vi "Main_v4_OJ.vi"() -> ()   [LabVIEW 2023]
uses:
  AD2_MSO_SDK_class/MSOConfig.ctl
  AD2_MSO_SDK_class/AD2TriggerSources.ctl
  AD2_MSO_SDK_class/MSORangeCh.ctl
  AD2_DO_SDK_class/DOConfigureCustomData.ctl
  AD2_DO_SDK_class/DOTrigger.ctl
  AD2_WFG_SDK_class/AD2TriggerSources.ctl
  AD2_DO_SDK_class/DOCustomData.ctl
  Application_class/Application.lvclass
  <vilib>/Utility/error.llb/Error Cluster From Error Code.vi
  <vilib>/ErrorRing/Error Ring.xnode
  AD2_SDK_class/AD2_SDK.lvclass
  AFG3022B_OJ_class/AFG3022B_OJ.lvclass
  Experiment_class/Experiment.lvclass
  TDMSLogger__class/TDMSLogger_class/TDMSLogger.lvclass
  CetoniPump_class/CetoniPump.lvclass
  TBS2000Series_class/TBS2000Series.lvclass
  TC0608_class/TC0608.lvclass
  AD2_DO_SDK_class/AD2_DO_SDK.lvclass
  AD2_MSO_SDK_class/AD2_MSO_SDK.lvclass
panel:
  out "Pump Status":T1(array[cluster])
  in  "Tab Control":T2(tab)=enum."InstrumentTests"
  in  "Cetoni Pump":bool
  in  "Initialize selected Instruments":bool
  in  "Peltier Controller":bool
  in  "Analog Discovery":bool
  in  "Function Generator":bool
  in  "Device Configuration Folder":string="C:\\Users\\Public\\Documents\\QmixElements\\Projects\\default_project\\Configurations\\sinle"
  in  "Peltier VISA resource name":refnum<visa-resource-name>
  in  "VISA resource name":refnum<visa-resource-name>
  in  "Change Freq Ch1 (Hz)":dbl
  in  "Enable Channels":cluster{"Ch1":bool, "Ch2":bool}
  in  "Oscilloscope Test":cluster{"Source Main":i32, "Source Probe":i32}={"Source Main"=2, "Source Probe"=1} {"Source Probe" items=["Math", "Channel 1", "Channel 2", "Channel 3", "Channel 4"]; "Source Main" items=["Math", "Channel 1", "Channel 2", "Channel 3", "Channel 4"]}
  in  "ReadOscilloscopeChannel":bool
  out "Temperature (C)":dbl
  in  "Read Peltier":bool
  in  "Image  Aquisition":T3={"Minimum Time between frames(s)"=10.0, "Number of Frames"=0} {"Minimum Time between frames(s)" min=0.005}
  in  "Take Images":bool
  in  "Pump: GoToLevel":bool
  in  "GoToLevelSettings":T4
  in  "refill below level":dbl=1000.0
  in  "Timeout Refill":dbl=20.0 caption="Time Target (s)"
  in  "Pump: CheckLevel&Refill":bool
  in  "Pump: Reference Move":bool
  in  "Pump: Refill":bool
  in  "Index":i32
  in  "Pump: Empty":bool
  in  "Pump: Read Status":bool
  in  "SyringeSettings":T5={"Maximum Piston Stroke (mm)"=100.0, "Inner Diameter (mm)"=12.0}
  in  "index configure syringe":i32
  in  "Pump: Configure":bool
  in  "Pump: STOP":bool
  in  "Source (1: Channel 1)":i32(ring)=1 items=["Math", "Channel 1", "Channel 2", "Channel 3", "Channel 4"]
  out "Peak-to-Peak":dbl format="%.2p"
  out "Frequency":dbl format="%.2p"
  in  "MeasurePowerOsc":bool
  out "Oscilloscope Results Test":T6 {"Probe Current" format="%.2p"; "Phase Angle" format="%.2p"; "Main Freq" format="%.2p"; "Main Volt" format="%.2p"}
  in  "milliseconds to wait 2":u32
  in  "Refill Rate(ul/min)":dbl=10000.0
  in  "Function Generator":T7
  in  "Change Amplitude Ch1(V)":dbl min=0.0 max=10.0
  in  "Wait After cond Refill":dbl
  in  "Start Experiment":bool
  in  "List of Frequencies":dbl[](array[numeric]) min=0.001
  in  "List of Amplitudes":dbl[](array[numeric]) min=0.001
  in  "List of Flow rates":dbl[](array[numeric])
  out "Total Number of Commands in Experiment":i32
  out "Commands Left in Experiment":i32
  out "Experiment Progress (%)":dbl
  in  "Number of Images at each frequency":i32
  in  "wait after frequency change (s)":dbl
  in  "wait between frames (s)":dbl
  in  "Freq Start":dbl
  in  "Freq Increment":dbl
  in  "Number of Frequencies":i32
  in  "FIll Frequency List":bool
  out "LOG":string
  in  "Time To wait":dbl
  in  "Wait":bool
  in  "Configure MSO":bool
  in  "MSO":T8={"Timing"={"Enable"=TRUE, "Samples In"=100000.0, "Sample Rate"=1250000.0, "Mode"=enum."Single Sample"}, "Trigger"={"Hysteresis"=0.0, "Trigger Level"=0.0, "Trigger Condition"=0, "Trigger Type"=0, "Trigger Channel"=0, "secTimeout"=1.0, "TrigrSrc"=enum."trigrsrcNone"}, "Range Ch1"={"idxChannel"=0, "voltOffset"=0.0, "VoltsRange"=50}, "Range Ch 2"={"idxChannel"=1, "voltOffset"=0.0, "VoltsRange"=50}} {"Range Ch 2"."VoltsRange" items=["High 50V"=50, "Low5V"=5]; "Range Ch1"."VoltsRange" items=["High 50V"=50, "Low5V"=5]; "Trigger"."Trigger Channel" items=["Channel 1"=0, "Channel 2"=1, "Both"=-1]; "Trigger"."Trigger Type" items=["Edge", "Pulse", "Transition"]; "Trigger"."Trigger Condition" items=["Rising", "Falling"]}
  in  "Read MSO":bool
  out "Waveform Graph":waveform(dbl)[](graph)
  out "Power (W)":dbl format="%0.2p"
  out "Impedance":dbl
  out "Phase (deg)":dbl
  in  "MeasurePower":bool
  in  "Trigg AD2":bool
  in  "Configure DO":bool
  in  "?":T11={"DO Trigger"={"secRun(0=Cont)"=0.0, "secWait"=0.0, "cRepeat(0=inf)"=0, "Repeat Trigger"=TRUE, "TrigrSrc"=enum."trigsrcPC"}, "CustomData"=[{"Data"=[FALSE, TRUE, FALSE, FALSE, FALSE, FALSE, FALSE, FALSE, FALSE, FALSE, FALSE, FALSE, FALSE, FALSE, FALSE, FALSE, FALSE, FALSE, FALSE, FALSE, FALSE, FALSE], "Freq"=1000.0, "#Bits"=100, "Enable"=TRUE, "IdleState"=0}, {"Data"=[], "Freq"=0.0, "#Bits"=0, "Enable"=FALSE, "IdleState"=0}, {"Data"=[], "Freq"=0.0, "#Bits"=0, "Enable"=FALSE, "IdleState"=0}, {"Data"=[], "Freq"=0.0, "#Bits"=0, "Enable"=FALSE, "IdleState"=0}, {"Data"=[], "Freq"=0.0, "#Bits"=0, "Enable"=FALSE, "IdleState"=0}, {"Data"=[], "Freq"=0.0, "#Bits"=0, "Enable"=FALSE, "IdleState"=0}, {"Data"=[], "Freq"=0.0, "#Bits"=0, "Enable"=FALSE, "IdleState"=0}, {"Data"=[], "Freq"=0.0, "#Bits"=0, "Enable"=FALSE, "IdleState"=0}, {"Data"=[], "Freq"=0.0, "#Bits"=0, "Enable"=FALSE, "IdleState"=0}, {"Data"=[], "Freq"=0.0, "#Bits"=0, "Enable"=FALSE, "IdleState"=0}, {"Data"=[], "Freq"=0.0, "#Bits"=0, "Enable"=FALSE, "IdleState"=0}, {"Data"=[], "Freq"=0.0, "#Bits"=0, "Enable"=FALSE, "IdleState"=0}, {"Data"=[], "Freq"=0.0, "#Bits"=0, "Enable"=FALSE, "IdleState"=0}, {"Data"=[FALSE, FALSE, FALSE, FALSE, FALSE, FALSE, FALSE, FALSE, FALSE, FALSE, FALSE, FALSE, FALSE, FALSE, FALSE, FALSE, FALSE, FALSE, FALSE, FALSE, FALSE, FALSE, FALSE], "Freq"=0.0, "#Bits"=0, "Enable"=FALSE, "IdleState"=0}, {"Data"=[FALSE, FALSE, FALSE, FALSE, FALSE, FALSE, FALSE, FALSE, FALSE, FALSE, FALSE, FALSE, FALSE, FALSE, FALSE, FALSE, FALSE, FALSE, FALSE, FALSE, FALSE, FALSE, FALSE], "Freq"=0.0, "#Bits"=0, "Enable"=FALSE, "IdleState"=0}]}
  in  "ABORT":bool
  out "Status":string="Program Started\nPlease connect to instruments"
  out "error out":errorcluster
  in  "Exit":bool
  # "Notes: \nChange frequency input to MHz\ninvestigate index in GoToLevelSettings, might be unneccesary"
  # "Peltier"
  # "Camera"
  # "Pump"
  # "Function Generator"
  # "Oscilloscope"
  # "Choose this carefully!\nYou can probably set this one low, since reading the peltier is slow. You might get problems when you start streaming images to HDD.\nThe program doesnt know when the camera is ready to aquire a new image. For large experiments you cannot store all images in RAM"
  # "The Pump will use index 0 for experiments\nPlease put your syringe here"
  # "Change Flow Rate\nChange Amplitude\nChange Frequency\nConditional Refill and wait\nEnable FG ch1\nWait\nRecord N times\nDisable Ch1\nWait\nRecord N times"
  # "Connect Ch1 to Piezo\nConnect Ch2 to voltage probe\nSet VoltsRange to LOW on ch2"
  # "Not sure if this is needed if we read the oscilloscope manually instead"
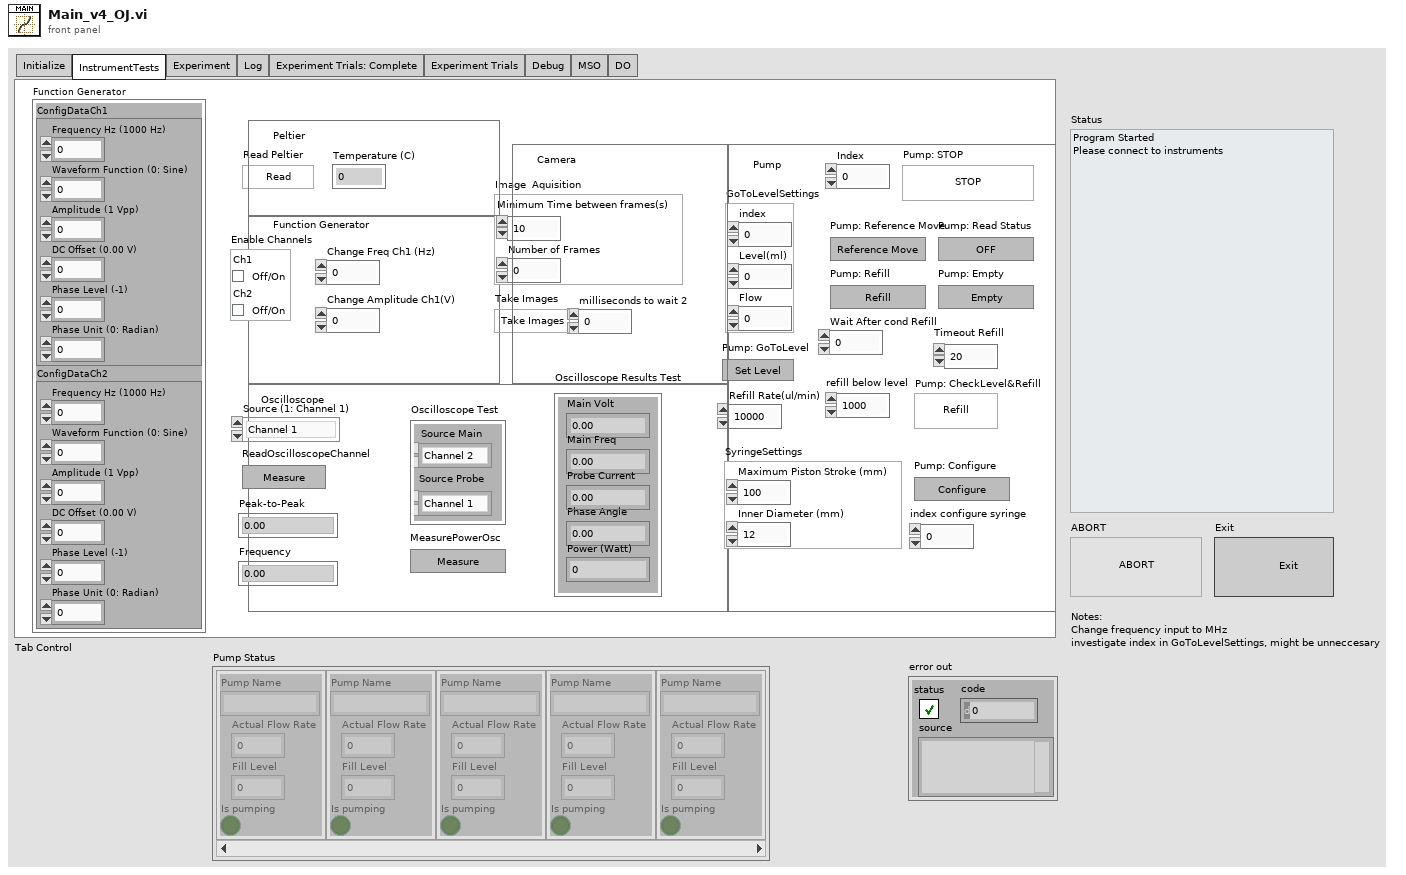
[diagram p1: front panel]
types:
  T1 = cluster{"Pump Name":string, "Actual Flow Rate":dbl, "Fill Level":dbl, "Is pumping":bool}[]
  T2 = enum32{"Initialize", "InstrumentTests", "Experiment", "Log", "Experiment Trials: Complete", "Experiment Trials", "Debug", "MSO", "DO"}
  T3 = cluster{"Minimum Time between frames(s)":dbl, "Number of Frames":i32}
  T4 = cluster{"index":i32, "Level(ml)":dbl, "Flow":dbl}
  T5 = cluster{"Maximum Piston Stroke (mm)":dbl, "Inner Diameter (mm)":dbl}
  T6 = cluster{"Main Volt":dbl, "Main Freq":dbl, "Phase Angle":dbl, "Probe Current":dbl, "Power (Watt)":dbl}
  T7 = cluster{"ConfigDataCh1":cluster{"Frequency Hz (1000 Hz)":dbl, "Waveform Function (0: Sine)":u16, "Amplitude (1 Vpp)":dbl, "DC Offset (0.00 V)":dbl, "Phase Level (-1)":dbl, "Phase Unit (0: Radian)":u16}, "ConfigDataCh2":cluster{"Frequency Hz (1000 Hz)":dbl, "Waveform Function (0: Sine)":u16, "Amplitude (1 Vpp)":dbl, "DC Offset (0.00 V)":dbl, "Phase Level (-1)":dbl, "Phase Unit (0: Radian)":u16}}
  T8 = typedef "AD2_MSO_SDK.lvclass/MSOConfig.ctl" = cluster{"Timing":cluster{"Enable":bool, "Samples In":dbl, "Sample Rate":dbl, "Mode":enum16{"Single Sample", "Scanshift", "Multiple Samples", "Scan Screen"}}, "Trigger":cluster{"Hysteresis":dbl, "Trigger Level":dbl, "Trigger Condition":i32, "Trigger Type":i32, "Trigger Channel":i32, "secTimeout":dbl, "TrigrSrc":T9}, "Range Ch1":T10, "Range Ch 2":T10}
  T9 = typedef "AD2_MSO_SDK.lvclass/AD2TriggerSources.ctl" = enum8{"trigrsrcNone", "trigsrcPC", "trigsrcDetectorAnalogIn", "trigsrcDetectorDigitalIn", "trigsrcAnalogIn", "trigsrcDigitalIn", "trigsrcDigitalOut", "trigsrcAnalogOut1", "trigsrcAnalogOut2", "trigsrcAnalogOut3", "trigsrcAnalogOut4", "trigsrcExternal1", "trigsrcExternal2", "trigsrcExternal3", "trigsrcExternal4", ""}
  T10 = typedef "AD2_MSO_SDK.lvclass/MSORangeCh.ctl" = cluster{"idxChannel":i32, "voltOffset":dbl, "VoltsRange":u16}
  T11 = typedef "DOConfigureCustomData.ctl" = cluster{"DO Trigger":T12, "CustomData":T14}
  T12 = typedef "AD2_DO_SDK.lvclass/DOTrigger.ctl" = cluster{"secRun(0=Cont)":dbl, "secWait":dbl, "cRepeat(0=inf)":i32, "Repeat Trigger":bool, "TrigrSrc":T13}
  T13 = typedef "AD2_SDK.lvclass/AD2TriggerSources.ctl" = enum8{"trigrsrcNone", "trigsrcPC", "trigsrcDetectorAnalogIn", "trigsrcDetectorDigitalIn", "trigsrcAnalogIn", "trigsrcDigitalIn", "trigsrcDigitalOut", "trigsrcAnalogOut1", "trigsrcAnalogOut2", "trigsrcAnalogOut3", "trigsrcAnalogOut4", "trigsrcExternal1", "trigsrcExternal2", "trigsrcExternal3", "trigsrcExternal4", ""}
  T14 = typedef "AD2_DO_SDK.lvclass/DOCustomData.ctl" = cluster{"Data":bool[], "Freq":dbl, "#Bits":u32, "Enable":bool, "IdleState":u16}[]
  T15 = cluster{"Minimum Time between frames":dbl, "Number of Frames":i32}
  T16 = cluster{"Pump Handle":i64, "Pump Name":string, "Maximum Volume":dbl, "Maximum Flow Rate":dbl, "Flow Rate":dbl, "Target Level":dbl, "Valve Handle":i64, "Has Valve?":bool, "Actual valve position":i32}[]
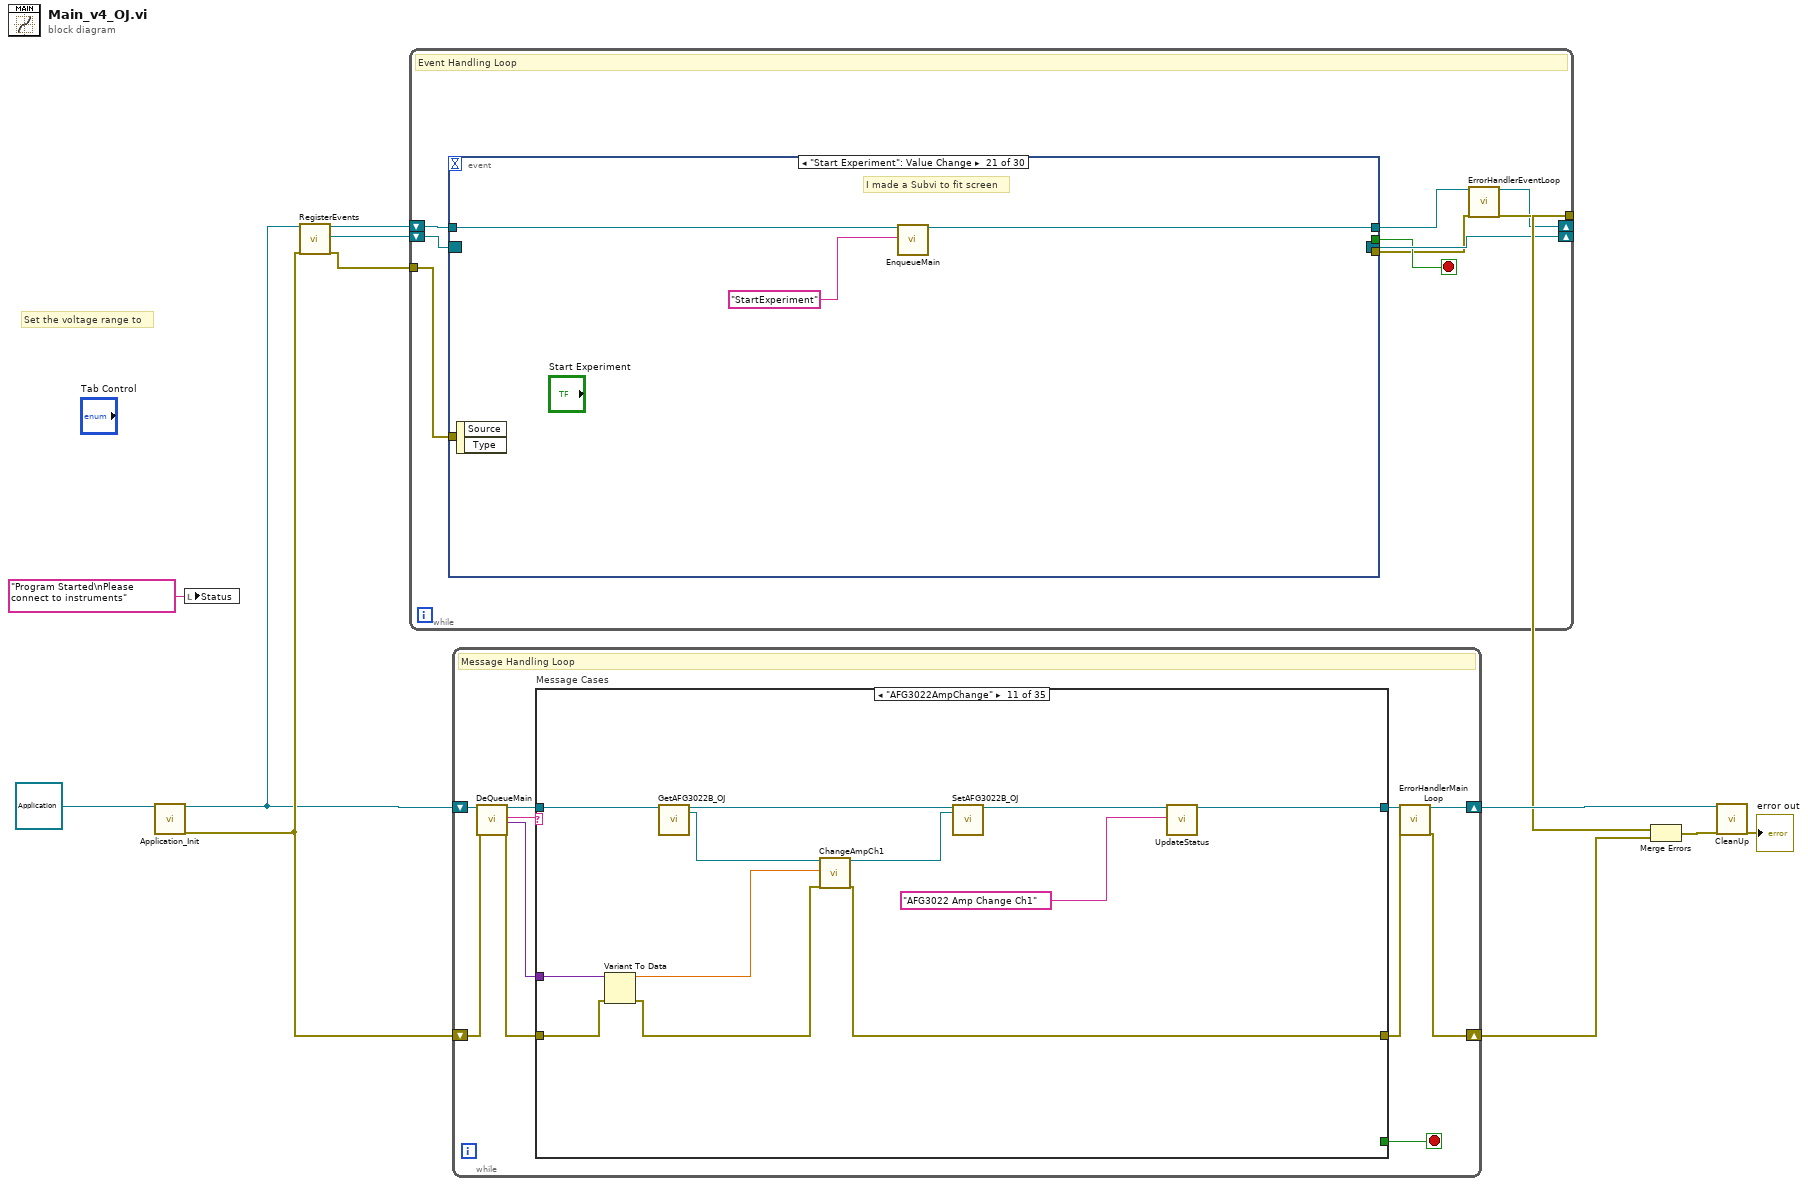
[diagram p0: block diagram]
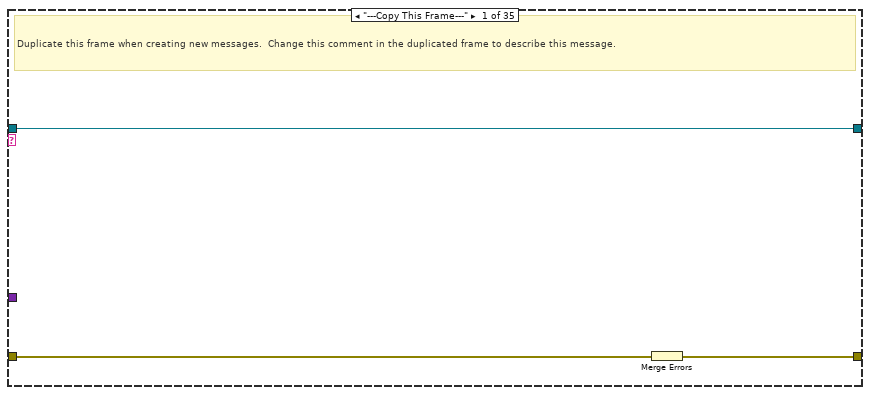
[diagram p2: hidden frame]
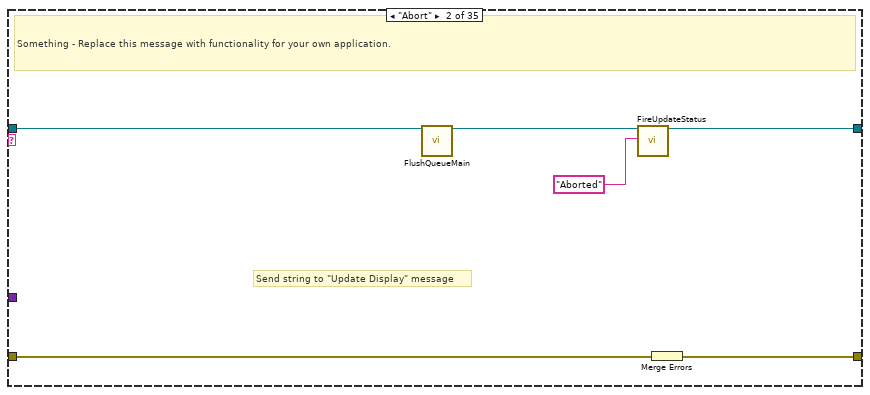
[diagram p3: hidden frame]
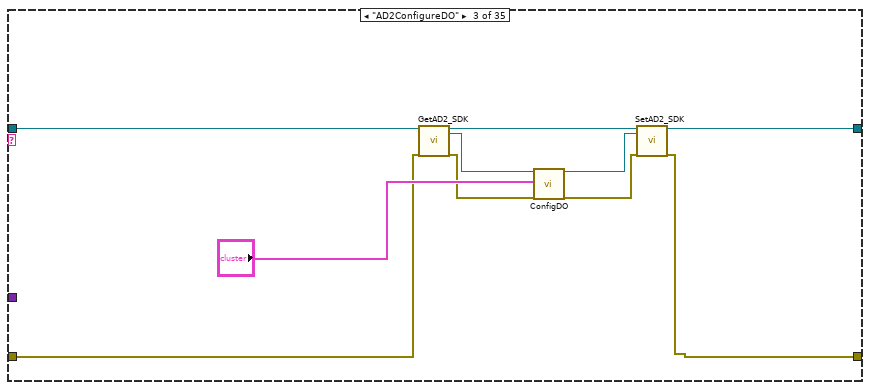
[diagram p4: hidden frame]
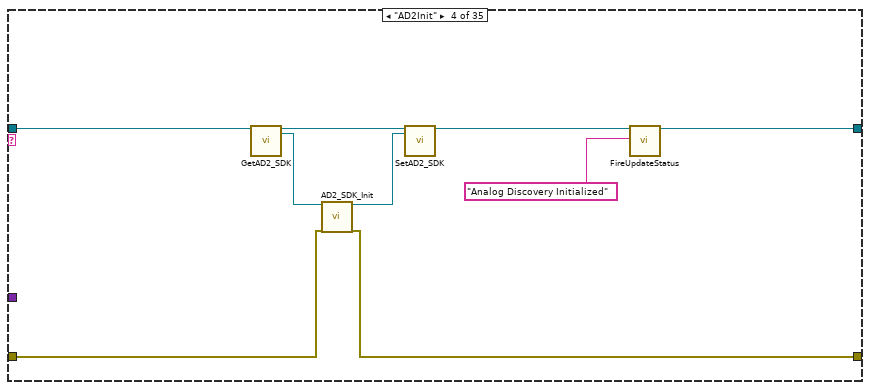
[diagram p5: hidden frame]
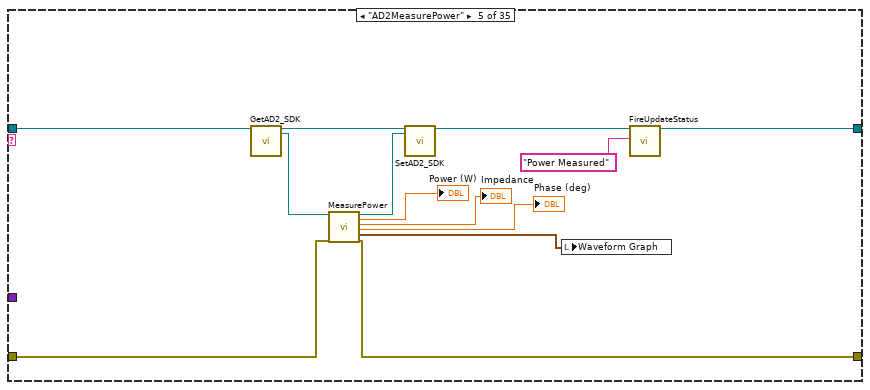
[diagram p6: hidden frame]
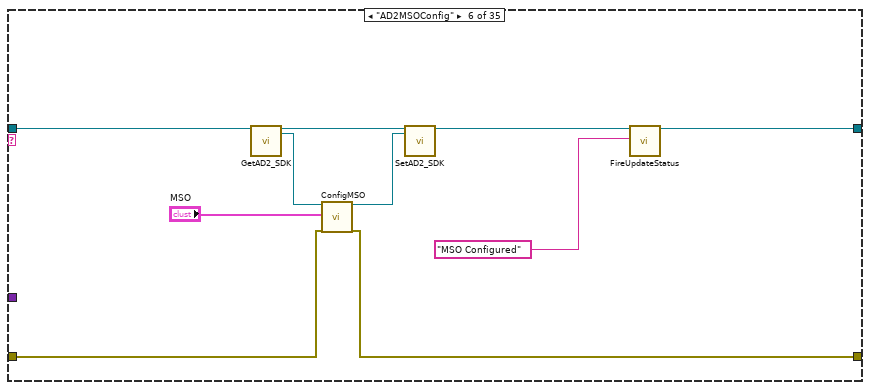
[diagram p7: hidden frame]
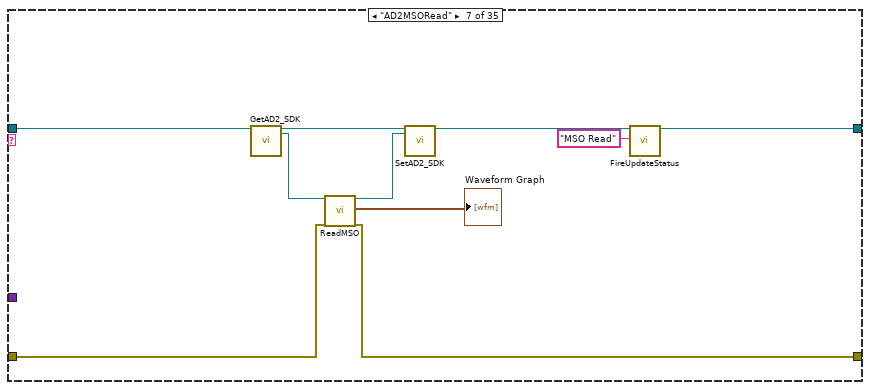
[diagram p8: hidden frame]
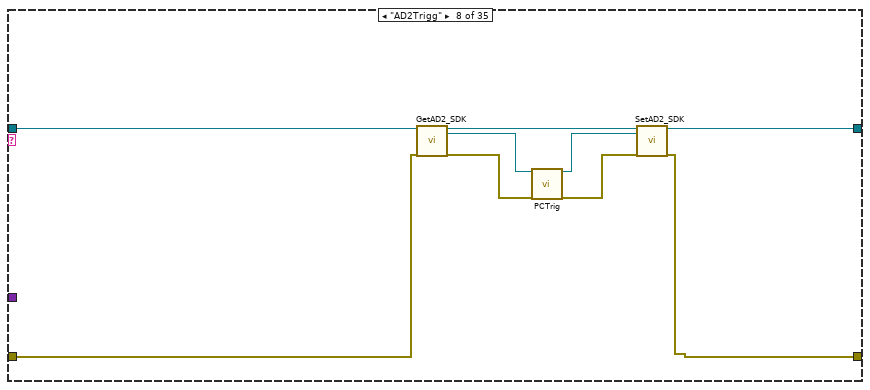
[diagram p9: hidden frame]
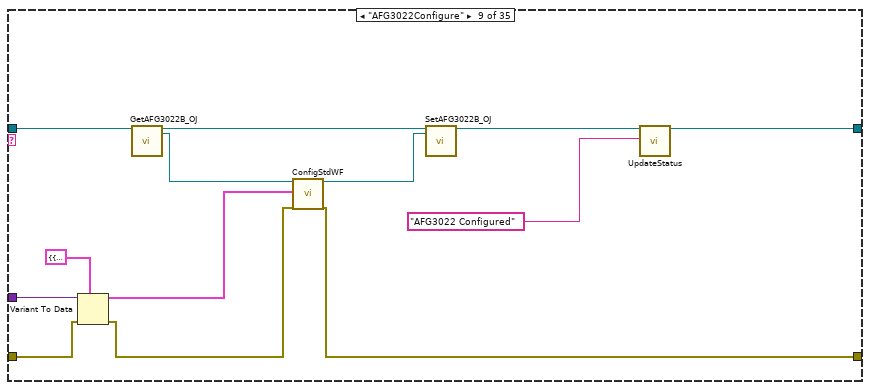
[diagram p10: hidden frame]
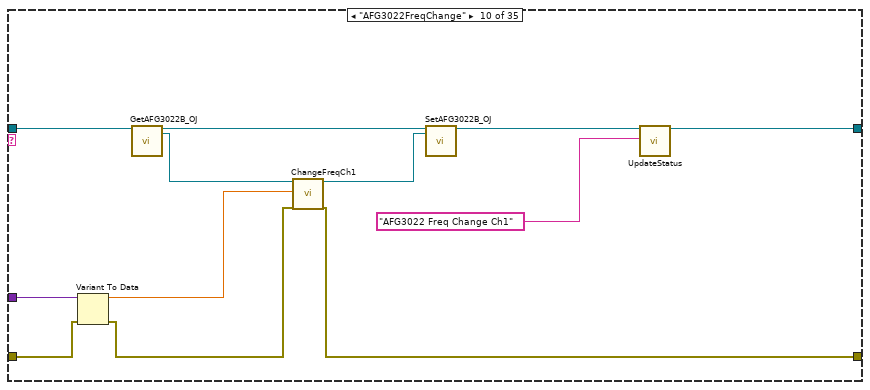
[diagram p11: hidden frame]
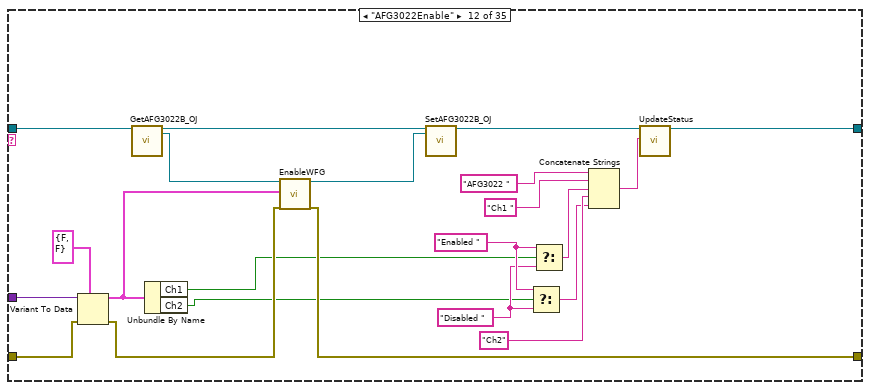
[diagram p12: hidden frame]
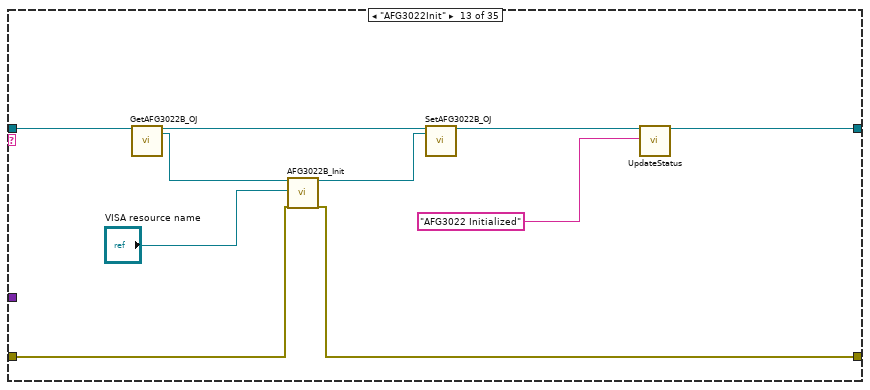
[diagram p13: hidden frame]
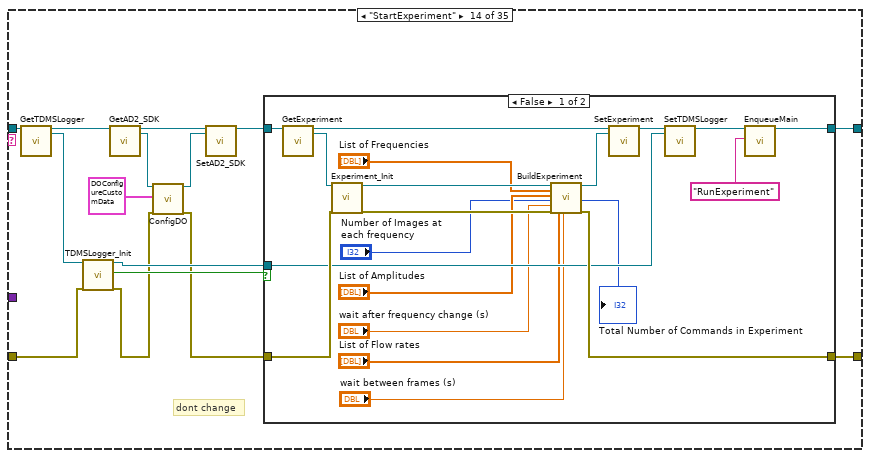
[diagram p14: hidden frame]
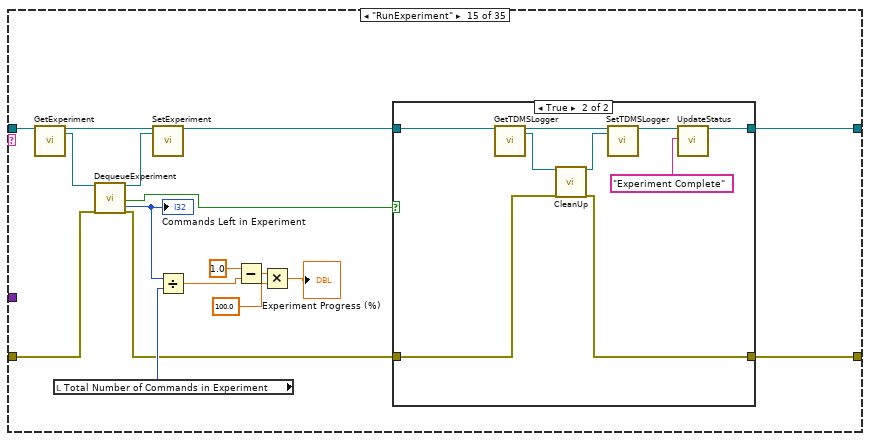
[diagram p16: hidden frame]
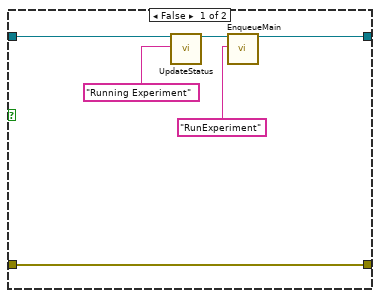
[diagram p17: hidden frame]
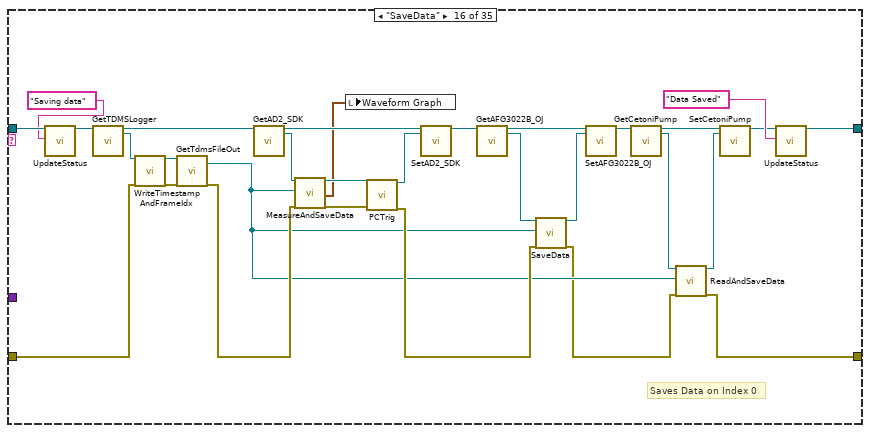
[diagram p18: hidden frame]
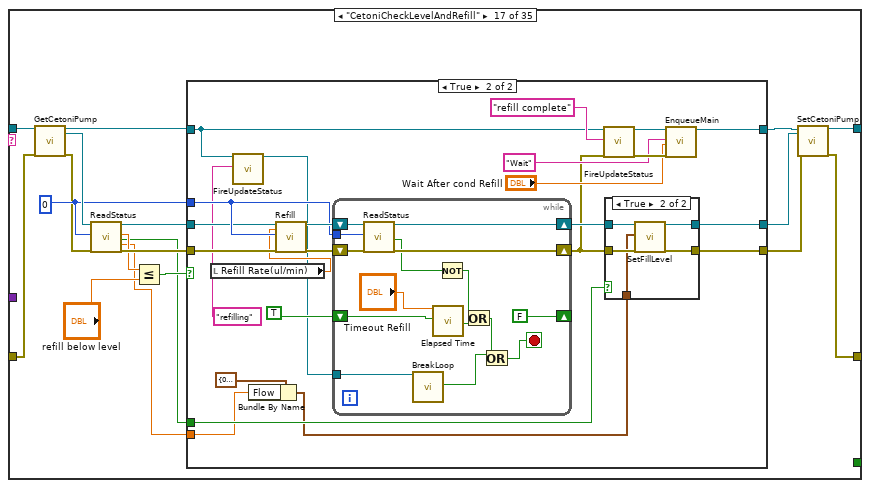
[diagram p19: hidden frame]
diagram:
  # "Set the voltage range to"
  n1 = call "Application_Init.vi"("object in"=refnum<class "Application.lvclass"> refnum ("Application")) -> ("object out"=w2:refnum<class "Application.lvclass">, "error out"=w8:errorcluster)  [unwired: 17 in]
  n2 = local write "Status"("Program Started\nPlease connect to instruments" ("Status")) -> ()
  n3 = call-dynamic "RegisterEvents.vi"("object in"=w2, "error in (no error)"=w8) -> ("object out"=w10:refnum<class "Application.lvclass">, "Event Registration Refnum"=w11:refnum<event-registration>, "error out"=w9:errorcluster)  [unwired: 15 in]
  n4 = while {
    shift-right: [w20] -> _
    shift-left: w11 -> [w21]
    tunnel: [w15] -> w5
    shift-right: [w13] -> _
    shift-left: w10 -> [w18]
    tunnel: w9 -> [w17]
    stop <- w19 stop-if-true
    # "Event Handling Loop"
    n5 = event shown="[20] \"Start Experiment\": Value Change" {
      selector: w21 -> [_ _ _ _ _ _ _ _ _ _ _ _ _ _ _ _ _ _ _ _ _ _ _ _ _ _ _ _ _ _]
      dyn-events: [_ _ _ _ _ _ _ _ _ _ _ _ _ _ _ _ _ _ _ _ _ _ _ _ _ _ _ _ _ _] -> w20
      timeout: _ -> [_ _ _ _ _ _ _ _ _ _ _ _ _ _ _ _ _ _ _ _ _ _ _ _ _ _ _ _ _ _]
      tunnel: [TRUE ("Discard?") _ _ _ _ _ _ _ _ _ _ _ _ _ _ _ _ _ _ _ _ _ _ _ _ _ _ _ _ _] -> w19
      tunnel: [w23 w29 w37 w42 _ _ _ w61 _ _ _ _ w95 w101 w107 w113 w118 w125 _ _ _ _ _ _ _ _ _ w165 _ _] -> w16
      tunnel: w18 -> [w28 w34 w36 w43 w47 w52 w60 w65 w77 w87 w89 w93 w96 w102 w108 w114 w119 w126 w137 w140 w143 w147 w151 w154 w157 w160 w163 w168 w185 w189]
      tunnel: [w27 w33 w35 w43 w46 w52 w59 w64 w76 w87 w89 w92 w97 w103 w109 w115 w120 w127 w136 w139 w142 w146 w150 w153 w156 w159 w162 w168 w184 w188] -> w14
      tunnel: w17 -> [w24 w30 w38 w42 _ _ _ w62 _ _ _ _ w94 w100 w106 w112 w117 w124 _ _ _ _ _ _ _ _ _ w166 _ _]
      event "Exit": Value Change {
        (unwired) "\"Exit\" button pressed" ("VI Stopped")
        n6 = event-data() -> ()  [unwired: 1 in, 1 out]
        n7 = call-dynamic "EnqueueMain.vi"("object in"=w28, "Message"="Exit", "error in (no error)"=w24, "Priority Message? (F)"=TRUE) -> ("object out"=w27:refnum<class "Application.lvclass">, "error out"=w23:errorcluster)  [unwired: 14 in]
      }
      event "ABORT": Value Change {
        n8 = event-data() -> ()  [unwired: 1 in, 1 out]
        n9 = call-dynamic "EnqueueMain.vi"("object in"=w34, "Message"="Abort", "error in (no error)"=w30, "Priority Message? (F)"=TRUE) -> ("object out"=w33:refnum<class "Application.lvclass">, "error out"=w29:errorcluster)  [unwired: 14 in]
      }
      event Panel Close? {
        # "Send the 'Confirm Quit' message if the user closes the panel of the VI. Discard the event so the 'Confirm Quit' message has a chance to run."
        n10 = event-data() -> ()  [unwired: 1 in, 1 out]
        n11 = call-dynamic "EnqueueMain.vi"("object in"=w36, "Message"="Confirm Quit", "error in (no error)"=w38, "Priority Message? (F)"=TRUE) -> ("object out"=w35:refnum<class "Application.lvclass">, "error out"=w37:errorcluster)  [unwired: 14 in]
        n12 = event-data("Discard?"=TRUE) -> ()  [unwired: 1 in, 1 out]
      }
      event Application Instance Close {
        # "stop the pumps if it's not automatically build into the cetoni software\nsave the log to a file"
        # "#CodeRecommended - When a project closes, all VIs within that project are aborted and leave memory. However, any code placed in this event frame is guaranteed to run to completion, so add any cleanup code that absolutely must happen here."
        n13 = event-data() -> ()  [unwired: 1 in, 1 out]
      }
      event "Wait": Value Change {
        n14 = event-data() -> ()  [unwired: 1 in, 2 out]
        n15 = call-dynamic "EnqueueMain.vi"("object in"=w47, "Message"="Wait", "Message Data"="Time To wait") -> ("object out"=w46:refnum<class "Application.lvclass">)  [unwired: 15 in, 1 out]
      }
      event "FIll Frequency List": Value Change {
        n16 = event-data() -> ()  [unwired: 1 in, 6 out]
        n17 = for {
          N: "Number of Frequencies" -> [_]
          tunnel: "Freq Increment" -> [w56]
          tunnel: "Freq Start" -> [w54]
          tunnel: [w53] -> w48 mode=indexing
          i -> [w57]
          n18 = Multiply(x=w56, y=w57) -> (x*y=w55:dbl)
          n19 = Add(x=w54, y=w55) -> (x+y=w53:dbl)
        }
        n20 = local write "List of Frequencies"(w48) -> ()
      }
      event "MeasurePower": Value Change {
        n21 = event-data() -> ()  [unwired: 1 in, 2 out]
        n22 = call-dynamic "EnqueueMain.vi"("object in"=w60, "Message"="AD2MeasurePower") -> ("object out"=w59:refnum<class "Application.lvclass">)  [unwired: 16 in, 1 out]
      }
      event "Read Peltier": Value Change {
        n23 = event-data() -> ()  [unwired: 1 in, 2 out]
        n24 = call-dynamic "EnqueueMain.vi"("object in"=w65, "Message"="PeltierRead", "error in (no error)"=w62) -> ("object out"=w64:refnum<class "Application.lvclass">, "error out"=w61:errorcluster)  [unwired: 15 in]
      }
      event "Initialize selected Instruments": Value Change {
        n25 = event-data() -> ()  [unwired: 1 in, 6 out]
        n26 = Build Array("AFG3022Init" ("Message"), "PeltierInit" ("Message"), "AD2Init" ("Message"), "CetoniInit" ("Message")) -> (w66:string[])
        n27 = Build Array("Function Generator", "Peltier Controller", "Analog Discovery", "Cetoni Pump") -> (w67:bool[])
        n28 = for {
          shift-right: [w80] -> w76
          shift-left: w77 -> [w81]
          tunnel: w67 -> [w79] mode=indexing
          tunnel: w66 -> [w78] mode=indexing
          n29 = case shown="False" w79 {
            tunnel: w81 -> [w82 w85]
            tunnel: [w82 w84] -> w80
            tunnel: w78 -> [_ w83]
            frame False {
            }
            frame True {
              n30 = call-dynamic "EnqueueMain.vi"("object in"=w85, "Message"=w83) -> ("object out"=w84:refnum<class "Application.lvclass">)  [unwired: 16 in, 1 out]
            }
          }
        }
      }
      event "MeasurePowerOsc": Value Change {
        n31 = event-data() -> ()  [unwired: 1 in, 2 out]
        n32 = call-dynamic "EnqueueMain.vi"("object in"=w87, "Message"="MeasurePowerOsc") -> ()  [unwired: 16 in, 2 out]
      }
      event "ReadOscilloscopeChannel": Value Change {
        n33 = event-data() -> ()  [unwired: 1 in, 2 out]
        n34 = call-dynamic "EnqueueMain.vi"("object in"=w89, "Message"="ReadOscilloscopeChannel") -> ()  [unwired: 16 in, 2 out]
      }
      event "Take Images": Value Change {
        n35 = event-data() -> ()  [unwired: 1 in, 2 out]
        n36 = call-dynamic "EnqueueMain.vi"("object in"=w93, "Message"="TakeNImages", "Message Data"="Image  Aquisition") -> ("object out"=w92:refnum<class "Application.lvclass">)  [unwired: 15 in, 1 out]
      }
      event "Pump: Configure": Value Change {
        n37 = event-data() -> ()  [unwired: 1 in, 2 out]
        n38 = call-dynamic "EnqueueMain.vi"("object in"=w96, "Message"="CetoniConfigureSyringe", "error in (no error)"=w94) -> ("object out"=w97:refnum<class "Application.lvclass">, "error out"=w95:errorcluster)  [unwired: 15 in]
      }
      event "Pump: GoToLevel": Value Change {
        n39 = event-data() -> ()  [unwired: 1 in, 2 out]
        n40 = call-dynamic "EnqueueMain.vi"("object in"=w102, "Message"="CetoniGoToLevel", "Message Data"="GoToLevelSettings", "error in (no error)"=w100) -> ("object out"=w103:refnum<class "Application.lvclass">, "error out"=w101:errorcluster)  [unwired: 14 in]
      }
      event "Pump: Empty": Value Change {
        n41 = event-data() -> ()  [unwired: 1 in, 2 out]
        n42 = local read "Index"() -> (w105:i32)
        n43 = call-dynamic "EnqueueMain.vi"("object in"=w108, "Message"="CetoniEmpty", "Message Data"=w105, "error in (no error)"=w106) -> ("object out"=w109:refnum<class "Application.lvclass">, "error out"=w107:errorcluster)  [unwired: 14 in]
      }
      event "Pump: Refill": Value Change {
        n44 = event-data() -> ()  [unwired: 1 in, 2 out]
        n45 = call-dynamic "EnqueueMain.vi"("object in"=w114, "Message"="CetoniRefill", "Message Data"="Index", "error in (no error)"=w112) -> ("object out"=w115:refnum<class "Application.lvclass">, "error out"=w113:errorcluster)  [unwired: 14 in]
      }
      event "Pump: Read Status": Value Change {
        n46 = event-data() -> ()  [unwired: 1 in, 2 out]
        n47 = call-dynamic "EnqueueMain.vi"("object in"=w119, "Message"="CetoniReadStatus", "error in (no error)"=w117) -> ("object out"=w120:refnum<class "Application.lvclass">, "error out"=w118:errorcluster)  [unwired: 15 in]
      }
      event "Pump: Reference Move": Value Change {
        n48 = event-data() -> ()  [unwired: 1 in, 2 out]
        n49 = Two Button Dialog(message="The pumps will perform a reference move. Please remove all syringes!!!!! ") -> (T button?=w123:bool)  [unwired: 2 in]
        n50 = case shown="True" w123 {
          tunnel: [w128 w133] -> w127
          tunnel: w126 -> [w128 w132]
          tunnel: [w129 w131] -> w125
          tunnel: w124 -> [w129 w130]
          frame False {
          }
          frame True {
            n51 = call-dynamic "EnqueueMain.vi"("object in"=w132, "Message"="CetoniReferenceMove", "error in (no error)"=w130) -> ("object out"=w133:refnum<class "Application.lvclass">, "error out"=w131:errorcluster)  [unwired: 15 in]
          }
        }
      }
      event "Pump: CheckLevel&Refill": Value Change {
        n52 = event-data() -> ()  [unwired: 1 in, 2 out]
        n53 = call-dynamic "EnqueueMain.vi"("object in"=w137, "Message"="CetoniCheckLevelAndRefill") -> ("object out"=w136:refnum<class "Application.lvclass">)  [unwired: 16 in, 1 out]
      }
      event "Pump: STOP": Value Change {
        n54 = event-data() -> ()  [unwired: 1 in, 1 out]
        n55 = call-dynamic "EnqueueMain.vi"("object in"=w140, "Message"="CetoniStopPumps") -> ("object out"=w139:refnum<class "Application.lvclass">)  [unwired: 16 in, 1 out]
      }
      event "Start Experiment": Value Change {
        # "I made a Subvi to fit screen"
        n56 = event-data() -> ()  [unwired: 1 in, 2 out]
        n57 = call-dynamic "EnqueueMain.vi"("object in"=w143, "Message"="StartExperiment") -> ("object out"=w142:refnum<class "Application.lvclass">)  [unwired: 16 in, 1 out]
      }
      event "Change Freq Ch1 (Hz)": Value Change {
        n58 = event-data() -> ()  [unwired: 1 in, 6 out]
        n59 = call-dynamic "EnqueueMain.vi"("object in"=w147, "Message"="AFG3022FreqChange", "Message Data"="Change Freq Ch1 (Hz)") -> ("object out"=w146:refnum<class "Application.lvclass">)  [unwired: 15 in, 1 out]
      }
      event "Change Amplitude Ch1(V)": Value Change {
        n60 = event-data() -> ()  [unwired: 1 in, 6 out]
        n61 = call-dynamic "EnqueueMain.vi"("object in"=w151, "Message"="AFG3022AmpChange", "Message Data"="Change Amplitude Ch1(V)") -> ("object out"=w150:refnum<class "Application.lvclass">)  [unwired: 15 in, 1 out]
      }
      event "Configure DO": Value Change {
        n62 = event-data() -> ()  [unwired: 1 in, 2 out]
        n63 = call-dynamic "EnqueueMain.vi"("object in"=w154, "Message"="AD2ConfigureDO") -> ("object out"=w153:refnum<class "Application.lvclass">)  [unwired: 16 in, 1 out]
      }
      event "Configure MSO": Value Change {
        n64 = event-data() -> ()  [unwired: 1 in, 2 out]
        n65 = call-dynamic "EnqueueMain.vi"("object in"=w157, "Message"="AD2MSOConfig") -> ("object out"=w156:refnum<class "Application.lvclass">)  [unwired: 16 in, 1 out]
      }
      event "Read MSO": Value Change {
        n66 = event-data() -> ()  [unwired: 1 in, 2 out]
        n67 = call-dynamic "EnqueueMain.vi"("object in"=w160, "Message"="AD2MSORead") -> ("object out"=w159:refnum<class "Application.lvclass">)  [unwired: 16 in, 1 out]
      }
      event "Trigg AD2": Value Change {
        n68 = event-data() -> ()  [unwired: 1 in, 2 out]
        n69 = call-dynamic "EnqueueMain.vi"("object in"=w163, "Message"="AD2Trigg") -> ("object out"=w162:refnum<class "Application.lvclass">)  [unwired: 16 in, 1 out]
      }
      event User Event {
        # "#tbd fix log"
        n70 = event-data() -> ("Message"=w167:string, "Message Data"=w164:variant)  [unwired: 1 in]
        n71 = case shown="\"UpdateStatus\"" w167 {
          tunnel: w166 -> [w172 w181]
          tunnel: [w172 w181] -> w165
          tunnel: w164 -> [w171 _]
          frame "UpdateStatus" {
            # "I have disabled the log, it might slow down the program\nwhen it becomes to large"
            n72 = Variant To Data(type="" ("Status"), Variant=w171) -> (data=w169:string)  [unwired: 1 in, 1 out]
            "Status" <- w169
            n73 = disable-structure shown="Disabled" {
              disable-tunnel: w169 -> [w176 _]
              frame Disabled {
                n74 = Get Date/Time In Seconds() -> (seconds since 1Jan1904=w180:timestamp)
                n75 = Get Date/Time String(seconds (now)=w180) -> (time string=w177:string)  [unwired: 2 in, 1 out]
                n76 = feedback #1("" ("string")) -> (w173:string)
                n77 = Concatenate Strings(w173, "\r", w177, "\t", w176) -> (w175:string)
                "LOG" <- w175
                n78 = feedback-in #1(w175) -> ()
              }
              frame Enabled {
              }
            }
          }
          frame Default {
          }
        }
      }
      event "Function Generator": Value Change {
        n79 = event-data() -> ()  [unwired: 1 in, 6 out]
        n80 = call-dynamic "EnqueueMain.vi"("object in"=w185, "Message"="AFG3022Configure", "Message Data"="Function Generator") -> ("object out"=w184:refnum<class "Application.lvclass">)  [unwired: 15 in, 1 out]
      }
      event "Enable Channels": Value Change {
        n81 = event-data() -> ()  [unwired: 1 in, 6 out]
        n82 = call-dynamic "EnqueueMain.vi"("object in"=w189, "Message"="AFG3022Enable", "Message Data"="Enable Channels") -> ("object out"=w188:refnum<class "Application.lvclass">)  [unwired: 15 in, 1 out]
      }
    }
    n83 = call-dynamic "ErrorHandlerEventLoop.vi"("object in"=w14, "error in (no error)"=w16) -> ("object out"=w13:refnum<class "Application.lvclass">, "error out"=w15:errorcluster)  [unwired: 16 in]
  }
  n84 = while {
    shift-right: [w193] -> w7
    shift-left: w2 -> [w199]
    shift-right: [w194] -> w6
    shift-left: w8 -> [w190]
    stop <- w200 stop-if-true
    # "Message Handling Loop"
    n85 = call-dynamic "DeQueueMain.vi"("object in"=w199, "error in (no error)"=w190) -> ("object out"=w198:refnum<class "Application.lvclass">, "Message"=w197:string, "Message Data"=w196:variant, "error out"=w191:errorcluster)  [unwired: 14 in]
    n86 = case "Message Cases" shown="\"AFG3022AmpChange\"" w197 {
      selector: w197 -> [_ _ _ _ _ _ _ _ _ _ _ _ _ _ _ _ _ _ _ _ _ _ _ _ _ _ _ _ _ _ _ _ _ _ w714]
      tunnel: w191 -> [w203 w208 w210 w224 w234 w247 w256 w266 w273 w285 w297 w324 w332 w347 w390 w427 w453 w512 w522 w533 w555 w566 w580 w596 w607 w618 w620 w634 w640 w650 w660 w674 w678 w710 _]
      tunnel: [w202 w209 w211 w225 w233 w248 w255 w267 w276 w288 w300 w320 w333 w353 w377 w413 w454 w514 w526 w542 w554 w568 w582 w600 w609 w613 w621 w634 w641 w651 w659 w674 w679 w706 w715] -> w195
      tunnel: [_ _ _ _ _ _ _ _ _ _ _ _ _ _ _ _ _ _ _ _ _ _ _ _ _ _ TRUE _ _ _ _ _ _ _ _] -> w200
      tunnel: w196 -> [_ _ _ _ _ _ _ _ w275 w287 w299 w325 _ _ _ _ _ _ w524 w535 _ _ _ w598 _ w617 _ _ _ _ _ _ w681 w712 _]
      tunnel: w198 -> [w201 w207 w219 w228 w241 w251 w261 w270 w282 w294 w306 w328 w337 w354 w393 w417 w456 w516 w528 w544 w556 w569 w584 w602 w611 w612 w622 w629 w647 w653 w663 w671 w685 w708 w713]
      tunnel: [w201 w205 w217 w221 w238 w243 w254 w268 w280 w292 w304 w326 w331 w352 w380 w420 w455 w515 w527 w543 w546 w558 w583 w601 w610 w612 w623 w630 w645 w649 w664 w672 w686 w703 w713] -> w192
      frame "---Copy This Frame---" {
        # "Duplicate this frame when creating new messages.  Change this comment in the duplicated frame to describe this message."
        n87 = Merge Errors(w203) -> (w202:errorcluster)
      }
      frame "Abort" {
        # "Send string to \"Update Display\" message"
        # "Something - Replace this message with functionality for your own application."
        n88 = call-dynamic "FlushQueueMain.vi"("object in"=w207) -> ("object out"=w206:refnum<class "Application.lvclass">)  [unwired: 16 in, 2 out]
        n89 = call-dynamic "FireUpdateStatus.vi"("object in"=w206, "Status"="Aborted") -> ("object out"=w205:refnum<class "Application.lvclass">)  [unwired: 16 in, 1 out]
        n90 = Merge Errors(w208) -> (w209:errorcluster)
      }
      frame "AD2ConfigureDO" {
        n91 = call-dynamic "GetAD2_SDK.vi"("object in"=w219, "error in (no error)"=w210) -> ("object out"=w218:refnum<class "Application.lvclass">, "AD2_SDK"=w215:refnum<class "AD2_SDK.lvclass">, "error out"=w214:errorcluster)  [unwired: 15 in]
        n92 = call-dynamic "ConfigDO.vi"("object in"=w215, 2:"?", "error in (no error)"=w214) -> ("object out"=w213:refnum<class "AD2_SDK.lvclass">, "error out"=w212:errorcluster)  [unwired: 15 in]
        n93 = call-dynamic "SetAD2_SDK.vi"("object in"=w218, "AD2_SDK"=w213, "error in (no error)"=w212) -> ("object out"=w217:refnum<class "Application.lvclass">, "error out"=w211:errorcluster)  [unwired: 15 in]
      }
      frame "AD2Init" {
        n94 = call-dynamic "GetAD2_SDK.vi"("object in"=w228) -> ("object out"=w227:refnum<class "Application.lvclass">, "AD2_SDK"=w223:refnum<class "AD2_SDK.lvclass">)  [unwired: 16 in, 1 out]
        n95 = call "AD2_SDK_Init.vi"("object in"=w223, "error in (no error)"=w224) -> ("object out"=w222:refnum<class "AD2_SDK.lvclass">, "error out"=w225:errorcluster)  [unwired: 16 in]
        n96 = call-dynamic "SetAD2_SDK.vi"("object in"=w227, "AD2_SDK"=w222) -> ("object out"=w226:refnum<class "Application.lvclass">)  [unwired: 16 in, 1 out]
        n97 = call-dynamic "FireUpdateStatus.vi"("object in"=w226, "Status"="Analog Discovery Initialized") -> ("object out"=w221:refnum<class "Application.lvclass">)  [unwired: 16 in, 1 out]
      }
      frame "AD2MeasurePower" {
        n98 = call-dynamic "GetAD2_SDK.vi"("object in"=w241) -> ("object out"=w240:refnum<class "Application.lvclass">, "AD2_SDK"=w236:refnum<class "AD2_SDK.lvclass">)  [unwired: 16 in, 1 out]
        n99 = call-dynamic "MeasurePower.vi"("object in"=w236, "error in (no error)"=w234) -> ("object out"=w235:refnum<class "AD2_SDK.lvclass">, "Power (W)"=→"Power (W)":dbl, "Impedance"=→"Impedance":dbl, "Phase (deg)"=→"Phase (deg)":dbl, "Channels array"=w229:waveform(dbl)[], "error out"=w233:errorcluster)  [unwired: 12 in]
        n100 = call-dynamic "SetAD2_SDK.vi"("object in"=w240, "AD2_SDK"=w235) -> ("object out"=w239:refnum<class "Application.lvclass">)  [unwired: 16 in, 1 out]
        n101 = local write "Waveform Graph"(w229) -> ()
        n102 = call-dynamic "FireUpdateStatus.vi"("object in"=w239, "Status"="Power Measured") -> ("object out"=w238:refnum<class "Application.lvclass">)  [unwired: 16 in, 1 out]
      }
      frame "AD2MSOConfig" {
        n103 = call-dynamic "GetAD2_SDK.vi"("object in"=w251) -> ("object out"=w250:refnum<class "Application.lvclass">, "AD2_SDK"=w246:refnum<class "AD2_SDK.lvclass">)  [unwired: 16 in, 1 out]
        n104 = call-dynamic "ConfigMSO.vi"("object in"=w246, "variant"="MSO", "error in (no error)"=w247) -> ("object out"=w245:refnum<class "AD2_SDK.lvclass">, "error out"=w248:errorcluster)  [unwired: 15 in]
        n105 = call-dynamic "SetAD2_SDK.vi"("object in"=w250, "AD2_SDK"=w245) -> ("object out"=w249:refnum<class "Application.lvclass">)  [unwired: 16 in, 1 out]
        n106 = call-dynamic "FireUpdateStatus.vi"("object in"=w249, "Status"="MSO Configured") -> ("object out"=w243:refnum<class "Application.lvclass">)  [unwired: 16 in, 1 out]
      }
      frame "AD2MSORead" {
        n107 = call-dynamic "GetAD2_SDK.vi"("object in"=w261) -> ("object out"=w260:refnum<class "Application.lvclass">, "AD2_SDK"=w258:refnum<class "AD2_SDK.lvclass">)  [unwired: 16 in, 1 out]
        n108 = call-dynamic "ReadMSO.vi"("object in"=w258, "error in (no error)"=w256) -> ("object out"=w257:refnum<class "AD2_SDK.lvclass">, "Channels array"=→"Waveform Graph":waveform(dbl)[], "error out"=w255:errorcluster)  [unwired: 15 in]
        n109 = call-dynamic "SetAD2_SDK.vi"("object in"=w260, "AD2_SDK"=w257) -> ("object out"=w259:refnum<class "Application.lvclass">)  [unwired: 16 in, 1 out]
        n110 = call-dynamic "FireUpdateStatus.vi"("object in"=w259, "Status"="MSO Read") -> ("object out"=w254:refnum<class "Application.lvclass">)  [unwired: 16 in, 1 out]
      }
      frame "AD2Trigg" {
        n111 = call-dynamic "GetAD2_SDK.vi"("object in"=w270, "error in (no error)"=w266) -> ("object out"=w269:refnum<class "Application.lvclass">, "AD2_SDK"=w265:refnum<class "AD2_SDK.lvclass">, "error out"=w263:errorcluster)  [unwired: 15 in]
        n112 = call-dynamic "PCTrig.vi"("object in"=w265, "error in (no error)"=w263) -> ("object out"=w264:refnum<class "AD2_SDK.lvclass">, "error out"=w262:errorcluster)  [unwired: 16 in]
        n113 = call-dynamic "SetAD2_SDK.vi"("object in"=w269, "AD2_SDK"=w264, "error in (no error)"=w262) -> ("object out"=w268:refnum<class "Application.lvclass">, "error out"=w267:errorcluster)  [unwired: 15 in]
      }
      frame "AFG3022Configure" {
        n114 = Variant To Data(error in=w273, type=T7 {"ConfigDataCh1"={"Frequency Hz (1000 Hz)"=1000.0, "Waveform Function (0: Sine)"=0, "Amplitude (1 Vpp)"=0.0, "DC Offset (0.00 V)"=0.0, "Phase Level (-1)"=0.0, "Phase Unit (0: Radian)"=0}, "ConfigDataCh2"={"Frequency Hz (1000 Hz)"=0.0, "Waveform Function (0: Sine)"=0, "Amplitude (1 Vpp)"=0.0, "DC Offset (0.00 V)"=0.0, "Phase Level (-1)"=0.0, "Phase Unit (0: Radian)"=0}} ("Function Generator"), Variant=w275) -> (data=w272:T7, error out=w274:errorcluster)
        n115 = call-dynamic "GetAFG3022B_OJ.vi"("object in"=w282) -> ("object out"=w281:refnum<class "Application.lvclass">, "AFG3022B_OJ"=w278:refnum<class "AFG3022B_OJ.lvclass">)  [unwired: 16 in, 1 out]
        n116 = call-dynamic "ConfigStdWF.vi"("object in"=w278, "Configdatastd"=w272, "error in (no error)"=w274) -> ("object out"=w277:refnum<class "AFG3022B_OJ.lvclass">, "error out"=w276:errorcluster)  [unwired: 15 in]
        n117 = call-dynamic "SetAFG3022B_OJ.vi"("object in"=w281, "AFG3022B_OJ"=w277) -> ("object out"=w283:refnum<class "Application.lvclass">)  [unwired: 16 in, 1 out]
        n118 = call-dynamic "UpdateStatus.vi"("object in"=w283, "Status"="AFG3022 Configured") -> ("object out"=w280:refnum<class "Application.lvclass">)  [unwired: 16 in, 1 out]
      }
      frame "AFG3022FreqChange" {
        n119 = Variant To Data(error in=w285, Variant=w287) -> (data=w284:dbl, error out=w286:errorcluster)  [unwired: 1 in]
        n120 = call-dynamic "GetAFG3022B_OJ.vi"("object in"=w294) -> ("object out"=w293:refnum<class "Application.lvclass">, "AFG3022B_OJ"=w290:refnum<class "AFG3022B_OJ.lvclass">)  [unwired: 16 in, 1 out]
        n121 = call-dynamic "ChangeFreqCh1.vi"("object in"=w290, "Frequency Hz (1000 Hz)"=w284, "error in (no error)"=w286) -> ("object out"=w289:refnum<class "AFG3022B_OJ.lvclass">, "error out"=w288:errorcluster)  [unwired: 15 in]
        n122 = call-dynamic "SetAFG3022B_OJ.vi"("object in"=w293, "AFG3022B_OJ"=w289) -> ("object out"=w295:refnum<class "Application.lvclass">)  [unwired: 16 in, 1 out]
        n123 = call-dynamic "UpdateStatus.vi"("object in"=w295, "Status"="AFG3022 Freq Change Ch1") -> ("object out"=w292:refnum<class "Application.lvclass">)  [unwired: 16 in, 1 out]
      }
      frame "AFG3022AmpChange" {
        n124 = Variant To Data(error in=w297, Variant=w299) -> (data=w296:dbl, error out=w298:errorcluster)  [unwired: 1 in]
        n125 = call-dynamic "GetAFG3022B_OJ.vi"("object in"=w306) -> ("object out"=w305:refnum<class "Application.lvclass">, "AFG3022B_OJ"=w302:refnum<class "AFG3022B_OJ.lvclass">)  [unwired: 16 in, 1 out]
        n126 = call-dynamic "ChangeAmpCh1.vi"("object in"=w302, "Amplitude (1 Vpp)"=w296, "error in (no error)"=w298) -> ("object out"=w301:refnum<class "AFG3022B_OJ.lvclass">, "error out"=w300:errorcluster)  [unwired: 15 in]
        n127 = call-dynamic "SetAFG3022B_OJ.vi"("object in"=w305, "AFG3022B_OJ"=w301) -> ("object out"=w307:refnum<class "Application.lvclass">)  [unwired: 16 in, 1 out]
        n128 = call-dynamic "UpdateStatus.vi"("object in"=w307, "Status"="AFG3022 Amp Change Ch1") -> ("object out"=w304:refnum<class "Application.lvclass">)  [unwired: 16 in, 1 out]
      }
      frame "AFG3022Enable" {
        w317 = "Disabled " ("Status")
        w318 = "Enabled " ("Status")
        n129 = Variant To Data(error in=w324, type=cluster{"Ch1":bool, "Ch2":bool} {"Ch1"=FALSE, "Ch2"=FALSE} ("Enable Channels"), Variant=w325) -> (data=w309:cluster{"Ch1":bool, "Ch2":bool}, error out=w321:errorcluster)
        n130 = call-dynamic "GetAFG3022B_OJ.vi"("object in"=w328) -> ("object out"=w327:refnum<class "Application.lvclass">, "AFG3022B_OJ"=w323:refnum<class "AFG3022B_OJ.lvclass">)  [unwired: 16 in, 1 out]
        n131 = Unbundle By Name(w309) -> ("Ch1"=w308:bool, "Ch2"=w316:bool)
        n132 = call-dynamic "EnableWFG.vi"("object in"=w323, "Enable Channels"=w309, "error in (no error)"=w321) -> ("object out"=w322:refnum<class "AFG3022B_OJ.lvclass">, "error out"=w320:errorcluster)  [unwired: 15 in]
        n133 = call-dynamic "SetAFG3022B_OJ.vi"("object in"=w327, "AFG3022B_OJ"=w322) -> ("object out"=w329:refnum<class "Application.lvclass">)  [unwired: 16 in, 1 out]
        n134 = Select(t=w318, s=w316, f=w317) -> (s? t:f=w310:string)
        n135 = Select(t=w318, s=w308, f=w317) -> (s? t:f=w312:string)
        n136 = Concatenate Strings("AFG3022 " ("Status"), "Ch1 " ("Status"), w312, "Ch2" ("Status"), w310) -> (w313:string)
        n137 = call-dynamic "UpdateStatus.vi"("object in"=w329, "Status"=w313) -> ("object out"=w326:refnum<class "Application.lvclass">)  [unwired: 16 in, 1 out]
      }
      frame "AFG3022Init" {
        n138 = call-dynamic "GetAFG3022B_OJ.vi"("object in"=w337) -> ("object out"=w336:refnum<class "Application.lvclass">, "AFG3022B_OJ"=w335:refnum<class "AFG3022B_OJ.lvclass">)  [unwired: 16 in, 1 out]
        n139 = call "AFG3022B_Init.vi"("object in"=w335, "VISA resource name"="VISA resource name", "error in (no error)"=w332) -> ("object out"=w334:refnum<class "AFG3022B_OJ.lvclass">, "error out"=w333:errorcluster)  [unwired: 15 in]
        n140 = call-dynamic "SetAFG3022B_OJ.vi"("object in"=w336, "AFG3022B_OJ"=w334) -> ("object out"=w338:refnum<class "Application.lvclass">)  [unwired: 16 in, 1 out]
        n141 = call-dynamic "UpdateStatus.vi"("object in"=w338, "Status"="AFG3022 Initialized") -> ("object out"=w331:refnum<class "Application.lvclass">)  [unwired: 16 in, 1 out]
      }
      frame "StartExperiment" {
        # "dont change"
        n142 = call-dynamic "GetTDMSLogger.vi"("object in"=w354) -> ("object out"=w351:refnum<class "Application.lvclass">, "TDMSLogger"=w350:refnum<class "TDMSLogger.lvclass">)  [unwired: 16 in, 1 out]
        n143 = call "TDMSLogger_Init.vi"("object in"=w350, "error in (no error)"=w347) -> ("object out"=w348:refnum<class "TDMSLogger.lvclass">, "cancelled"=w349:bool, "error out"=w341:errorcluster)  [unwired: 15 in]
        n144 = call-dynamic "GetAD2_SDK.vi"("object in"=w351) -> ("object out"=w346:refnum<class "Application.lvclass">, "AD2_SDK"=w343:refnum<class "AD2_SDK.lvclass">)  [unwired: 16 in, 1 out]
        n145 = call-dynamic "ConfigDO.vi"("object in"=w343, 2:T11 {"DO Trigger"={"secRun(0=Cont)"=0.005, "secWait"=0.0, "cRepeat(0=inf)"=0, "Repeat Trigger"=TRUE, "TrigrSrc"=enum."trigsrcPC"}, "CustomData"=[{"Data"=[FALSE, TRUE, FALSE, FALSE, FALSE, FALSE, FALSE, FALSE, FALSE, FALSE, FALSE, FALSE, FALSE, FALSE, FALSE, FALSE, FALSE, FALSE, FALSE, FALSE, FALSE, FALSE], "Freq"=1000.0, "#Bits"=100, "Enable"=TRUE, "IdleState"=0}, {"Data"=[], "Freq"=0.0, "#Bits"=0, "Enable"=FALSE, "IdleState"=0}, {"Data"=[], "Freq"=0.0, "#Bits"=0, "Enable"=FALSE, "IdleState"=0}, {"Data"=[], "Freq"=0.0, "#Bits"=0, "Enable"=FALSE, "IdleState"=0}, {"Data"=[], "Freq"=0.0, "#Bits"=0, "Enable"=FALSE, "IdleState"=0}, {"Data"=[], "Freq"=0.0, "#Bits"=0, "Enable"=FALSE, "IdleState"=0}, {"Data"=[], "Freq"=0.0, "#Bits"=0, "Enable"=FALSE, "IdleState"=0}, {"Data"=[], "Freq"=0.0, "#Bits"=0, "Enable"=FALSE, "IdleState"=0}, {"Data"=[], "Freq"=0.0, "#Bits"=0, "Enable"=FALSE, "IdleState"=0}, {"Data"=[], "Freq"=0.0, "#Bits"=0, "Enable"=FALSE, "IdleState"=0}, {"Data"=[], "Freq"=0.0, "#Bits"=0, "Enable"=FALSE, "IdleState"=0}, {"Data"=[], "Freq"=0.0, "#Bits"=0, "Enable"=FALSE, "IdleState"=0}, {"Data"=[], "Freq"=0.0, "#Bits"=0, "Enable"=FALSE, "IdleState"=0}]}, "error in (no error)"=w341) -> ("object out"=w342:refnum<class "AD2_SDK.lvclass">, "error out"=w340:errorcluster)  [unwired: 15 in]
        n146 = call-dynamic "SetAD2_SDK.vi"("object in"=w346, "AD2_SDK"=w342) -> ("object out"=w344:refnum<class "Application.lvclass">)  [unwired: 16 in, 1 out]
        n147 = case shown="False" w349 {
          tunnel: w340 -> [w371 w375]
          tunnel: [w367 w375] -> w353
          tunnel: [w357 w376] -> w352
          tunnel: w344 -> [w366 w376]
          tunnel: w348 -> [w365 _]
          frame False {
            n148 = call-dynamic "GetExperiment.vi"("object in"=w366) -> ("object out"=w373:refnum<class "Application.lvclass">, "Experiment"=w372:refnum<class "Experiment.lvclass">)  [unwired: 16 in, 1 out]
            n149 = call "Experiment_Init.vi"("object in"=w372, "error in (no error)"=w371) -> ("object out"=w370:refnum<class "Experiment.lvclass">, "error out"=w368:errorcluster)  [unwired: 16 in]
            n150 = call-dynamic "BuildExperiment.vi"("object in"=w370, "List of Frequencies"="List of Frequencies", "List of Amplitudes"="List of Amplitudes", "Number of Images at each frequency"="Number of Images at each frequency", "wait time(s)"="wait after frequency change (s)", "error in (no error)"=w368, "Flow"="List of Flow rates", "wait between frames"="wait between frames (s)") -> ("object out"=w369:refnum<class "Experiment.lvclass">, "# elements in queue"=→"Total Number of Commands in Experiment":i32, "error out"=w367:errorcluster)  [unwired: 9 in]
            n151 = call-dynamic "SetExperiment.vi"("object in"=w373, "Experiment"=w369) -> ("object out"=w374:refnum<class "Application.lvclass">)  [unwired: 16 in, 1 out]
            n152 = call-dynamic "SetTDMSLogger.vi"("object in"=w374, "TDMSLogger"=w365) -> ("object out"=w358:refnum<class "Application.lvclass">)  [unwired: 16 in, 1 out]
            n153 = call-dynamic "EnqueueMain.vi"("object in"=w358, "Message"="RunExperiment") -> ("object out"=w357:refnum<class "Application.lvclass">)  [unwired: 16 in, 1 out]
          }
          frame True {
          }
        }
      }
      frame "RunExperiment" {
        n154 = call-dynamic "GetExperiment.vi"("object in"=w393) -> ("object out"=w392:refnum<class "Application.lvclass">, "Experiment"=w391:refnum<class "Experiment.lvclass">)  [unwired: 16 in, 1 out]
        n155 = local read "Total Number of Commands in Experiment"() -> (w387:i32)
        n156 = call-dynamic "DequeueExperiment.vi"("object in"=w391, "error in (no error)"=w390) -> ("# elements in queue"=w388:i32, "object out"=w389:refnum<class "Experiment.lvclass">, "QueueEmpty"=w379:bool, "error out"=w378:errorcluster)  [unwired: 12 in, 2 out]
        "Commands Left in Experiment" <- w388
        n157 = call-dynamic "SetExperiment.vi"("object in"=w392, "Experiment"=w389) -> ("object out"=w381:refnum<class "Application.lvclass">)  [unwired: 16 in, 1 out]
        n158 = Divide(x=w388, y=w387) -> (x/y=w385:dbl)
        n159 = Subtract(x=1.0, y=w385) -> (x-y=w384:dbl)
        n160 = Multiply(x=w384, y=100.0) -> (x*y=→"Experiment Progress (%)":dbl)
        n161 = case shown="True" w379 {
          tunnel: w381 -> [w398 w408]
          tunnel: [w397 w401] -> w380
          tunnel: [w396 w404] -> w377
          tunnel: w378 -> [w396 w403]
          frame False {
            n162 = call-dynamic "UpdateStatus.vi"("object in"=w398, "Status"="Running Experiment") -> ("object out"=w395:refnum<class "Application.lvclass">)  [unwired: 16 in, 1 out]
            n163 = call-dynamic "EnqueueMain.vi"("object in"=w395, "Message"="RunExperiment") -> ("object out"=w397:refnum<class "Application.lvclass">)  [unwired: 16 in, 1 out]
          }
          frame True {
            n164 = call-dynamic "GetTDMSLogger.vi"("object in"=w408) -> ("object out"=w407:refnum<class "Application.lvclass">, "TDMSLogger"=w406:refnum<class "TDMSLogger.lvclass">)  [unwired: 16 in, 1 out]
            n165 = call-dynamic "CleanUp.vi"("object in"=w406, "error in (no error)"=w403) -> ("object out"=w405:refnum<class "TDMSLogger.lvclass">, "error out"=w404:errorcluster)  [unwired: 16 in]
            n166 = call-dynamic "SetTDMSLogger.vi"("object in"=w407, "TDMSLogger"=w405) -> ("object out"=w402:refnum<class "Application.lvclass">)  [unwired: 16 in, 1 out]
            n167 = call-dynamic "UpdateStatus.vi"("object in"=w402, "Status"="Experiment Complete") -> ("object out"=w401:refnum<class "Application.lvclass">)  [unwired: 16 in, 1 out]
          }
        }
      }
      frame "SaveData" {
        # "Saves Data on Index 0"
        n168 = call-dynamic "UpdateStatus.vi"("object in"=w417, "Status"="Saving data") -> ("object out"=w418:refnum<class "Application.lvclass">)  [unwired: 16 in, 1 out]
        n169 = call-dynamic "GetTDMSLogger.vi"("object in"=w418) -> ("object out"=w437:refnum<class "Application.lvclass">, "TDMSLogger"=w436:refnum<class "TDMSLogger.lvclass">)  [unwired: 16 in, 1 out]
        n170 = call-dynamic "WriteTimestampAndFrameIdx.vi"("object in"=w436, "error in (no error)"=w427) -> ("object out"=w435:refnum<class "TDMSLogger.lvclass">, "error out"=w429:errorcluster)  [unwired: 16 in]
        n171 = call-dynamic "GetTdmsFileOut.vi"("object in"=w435, "error in (no error)"=w429) -> ("tdms file out"=w415:refnum<k34>, "error out"=w428:errorcluster)  [unwired: 15 in, 1 out]
        n172 = call-dynamic "GetAD2_SDK.vi"("object in"=w437) -> ("object out"=w438:refnum<class "Application.lvclass">, "AD2_SDK"=w426:refnum<class "AD2_SDK.lvclass">)  [unwired: 16 in, 1 out]
        n173 = call-dynamic "MeasureAndSaveData.vi"("object in"=w426, "tdms file"=w415, "error in (no error)"=w428) -> ("object out"=w434:refnum<class "AD2_SDK.lvclass">, "Channels array"=w432:waveform(dbl)[], "error out"=w433:errorcluster)  [unwired: 14 in]
        n174 = local write "Waveform Graph"(w432) -> ()
        n175 = call-dynamic "PCTrig.vi"("object in"=w434, "error in (no error)"=w433) -> ("object out"=w430:refnum<class "AD2_SDK.lvclass">, "error out"=w421:errorcluster)  [unwired: 16 in]
        n176 = call-dynamic "SetAD2_SDK.vi"("object in"=w438, "AD2_SDK"=w430) -> ("object out"=w431:refnum<class "Application.lvclass">)  [unwired: 16 in, 1 out]
        n177 = call-dynamic "GetAFG3022B_OJ.vi"("object in"=w431) -> ("object out"=w425:refnum<class "Application.lvclass">, "AFG3022B_OJ"=w423:refnum<class "AFG3022B_OJ.lvclass">)  [unwired: 16 in, 1 out]
        n178 = call-dynamic "SaveData.vi"("object in"=w423, "tdms file"=w415, "error in (no error)"=w421) -> ("object out"=w422:refnum<class "AFG3022B_OJ.lvclass">, "error out"=w414:errorcluster)  [unwired: 15 in]
        n179 = call-dynamic "SetAFG3022B_OJ.vi"("object in"=w425, "AFG3022B_OJ"=w422) -> ("object out"=w424:refnum<class "Application.lvclass">)  [unwired: 16 in, 1 out]
        n180 = call-dynamic "GetCetoniPump.vi"("object in"=w424) -> ("object out"=w412:refnum<class "Application.lvclass">, "CetoniPump"=w410:refnum<class "CetoniPump.lvclass">)  [unwired: 16 in, 1 out]
        n181 = call-dynamic "ReadAndSaveData.vi"("object in"=w410, "tdms file"=w415, "error in (no error)"=w414) -> ("object out"=w409:refnum<class "CetoniPump.lvclass">, "error out"=w413:errorcluster)  [unwired: 15 in]
        n182 = call-dynamic "SetCetoniPump.vi"("object in"=w412, "CetoniPump"=w409) -> ("object out"=w411:refnum<class "Application.lvclass">)  [unwired: 16 in, 1 out]
        n183 = call-dynamic "UpdateStatus.vi"("object in"=w411, "Status"="Data Saved") -> ("object out"=w420:refnum<class "Application.lvclass">)  [unwired: 16 in, 1 out]
      }
      frame "CetoniCheckLevelAndRefill" {
        w451 = 0 ("index")
        n184 = call-dynamic "GetCetoniPump.vi"("object in"=w456, "error in (no error)"=w453) -> ("object out"=w442:refnum<class "Application.lvclass">, "CetoniPump"=w452:refnum<class "CetoniPump.lvclass">, "error out"=w444:errorcluster)  [unwired: 15 in]
        n185 = call-dynamic "ReadStatus.vi"("object in"=w452, "index"=w451, "error in (no error)"=w444) -> ("object out"=w450:refnum<class "CetoniPump.lvclass">, "Fill Level"=w447:dbl, "Is pumping"=w440:bool, "Actual Flow Rate"=w439:dbl, "error out"=w449:errorcluster)  [unwired: 12 in]
        n186 = Less Or Equal?(x=w447, y="refill below level") -> (x <= y?=w448:bool)
        n187 = case shown="True" w448 {
          tunnel: w451 -> [_ w482]
          tunnel: w450 -> [w459 w478]
          tunnel: w449 -> [w458 w480]
          tunnel: [w459 w466] -> w445
          tunnel: [w458 w460] -> w443
          tunnel: w442 -> [w457 w470]
          tunnel: [w457 w471] -> w441
          tunnel: w440 -> [_ w465]
          tunnel: w439 -> [_ w462]
          frame False {
          }
          frame True {
            n188 = local read "Refill Rate(ul/min)"() -> (w475:dbl)
            n189 = call-dynamic "FireUpdateStatus.vi"("object in"=w470, "Status"="refilling") -> ("object out"=w474:refnum<class "Application.lvclass">)  [unwired: 16 in, 1 out]
            n190 = Bundle By Name(cluster=T4 {"index"=0, "Level(ml)"=0.0, "Flow"=0.0} ("GoToLevelSettings"), "Flow"=w462) -> (w461:T4)
            n191 = call-dynamic "Refill.vi"("object in"=w478, "Refill Rate"=w475, "index"=w482, "error in (no error)"=w480) -> ("object out"=w483:refnum<class "CetoniPump.lvclass">, "error out"=w481:errorcluster)  [unwired: 14 in]
            n192 = while {
              tunnel: w482 -> [w504]
              shift-right: [w495] -> w467
              shift-left: w483 -> [w505]
              shift-right: [w502] -> w464
              shift-left: w481 -> [w503]
              shift-right: [FALSE] -> _
              shift-left: TRUE -> [w497]
              tunnel: w474 -> [w493]
              stop <- w491 stop-if-true
              n193 = call-dynamic "ReadStatus.vi"("object in"=w505, "index"=w504, "error in (no error)"=w503) -> ("object out"=w495:refnum<class "CetoniPump.lvclass">, "Is pumping"=w500:bool, "error out"=w502:errorcluster)  [unwired: 12 in, 2 out]
              n194 = call-dynamic "BreakLoop.vi"("object in"=w493) -> ("Abort"=w492:bool)  [unwired: 16 in, 2 out]
              n195 = call "Elapsed Time"("Time Target (s)"="Timeout Refill", "Reset"=w497) -> ("Time has Elapsed"=w498:bool)  [unwired: 10 in, 7 out]
              n196 = Not(x=w500) -> (.not. x?=w499:bool)
              n197 = Or(x=w499, y=w498) -> (x .or. y?=w494:bool)
              n198 = Or(x=w492, y=w494) -> (x .or. y?=w491:bool)
            }
            n199 = call-dynamic "FireUpdateStatus.vi"("object in"=w470, "Status"="refill complete", "error in (no error)"=w464) -> ("object out"=w472:refnum<class "Application.lvclass">, "error out"=w473:errorcluster)  [unwired: 15 in]
            n200 = case shown="True" w465 {
              tunnel: w467 -> [w485 w490]
              tunnel: [w485 w489] -> w466
              tunnel: w464 -> [w484 w488]
              tunnel: w461 -> [_ w487]
              tunnel: [w484 w486] -> w460
              frame False {
              }
              frame True {
                n201 = call-dynamic "SetFillLevel.vi"("object in"=w490, "GoToLevelSettings"=w487, "error in (no error)"=w488) -> ("object out"=w489:refnum<class "CetoniPump.lvclass">, "error out"=w486:errorcluster)  [unwired: 12 in, 3 out]
              }
            }
            n202 = call-dynamic "EnqueueMain.vi"("object in"=w472, "Message"="Wait" ("Status"), "Message Data"="Wait After cond Refill", "error in (no error)"=w473) -> ("object out"=w471:refnum<class "Application.lvclass">)  [unwired: 14 in, 1 out]
          }
        }
        n203 = call-dynamic "SetCetoniPump.vi"("object in"=w441, "CetoniPump"=w445, "error in (no error)"=w443) -> ("object out"=w455:refnum<class "Application.lvclass">, "error out"=w454:errorcluster)  [unwired: 15 in]
      }
      frame "CetoniConfigureSyringe" {
        n204 = call-dynamic "GetCetoniPump.vi"("object in"=w516, "error in (no error)"=w512) -> ("object out"=w513:refnum<class "Application.lvclass">, "CetoniPump"=w511:refnum<class "CetoniPump.lvclass">, "error out"=w507:errorcluster)  [unwired: 15 in]
        n205 = call-dynamic "ConfigureSyringe.vi"("object in"=w511, "index"="index configure syringe", "SyringeSettings"="SyringeSettings", "error in (no error)"=w507) -> ("object out"=w510:refnum<class "CetoniPump.lvclass">, "error out"=w506:errorcluster)  [unwired: 14 in]
        n206 = call-dynamic "SetCetoniPump.vi"("object in"=w513, "CetoniPump"=w510, "error in (no error)"=w506) -> ("object out"=w515:refnum<class "Application.lvclass">, "error out"=w514:errorcluster)  [unwired: 15 in]
      }
      frame "CetoniEmpty" {
        n207 = Variant To Data(error in=w522, Variant=w524) -> (data=w517:i32, error out=w523:errorcluster)  [unwired: 1 in]
        n208 = call-dynamic "GetCetoniPump.vi"("object in"=w528, "error in (no error)"=w523) -> ("object out"=w525:refnum<class "Application.lvclass">, "CetoniPump"=w521:refnum<class "CetoniPump.lvclass">, "error out"=w519:errorcluster)  [unwired: 15 in]
        n209 = call-dynamic "Empty.vi"("object in"=w521, "index"=w517, "error in (no error)"=w519) -> ("object out"=w520:refnum<class "CetoniPump.lvclass">, "error out"=w518:errorcluster)  [unwired: 15 in]
        n210 = call-dynamic "SetCetoniPump.vi"("object in"=w525, "CetoniPump"=w520, "error in (no error)"=w518) -> ("object out"=w527:refnum<class "Application.lvclass">, "error out"=w526:errorcluster)  [unwired: 15 in]
      }
      frame "CetoniGoToLevel" {
        # "Updates Control with coerced\nvalues"
        n211 = local read "GoToLevelSettings"() -> (w532:T4)
        n212 = Variant To Data(error in=w533, type=w532, Variant=w535) -> (data=w531:T4, error out=w534:errorcluster)
        n213 = call-dynamic "GetCetoniPump.vi"("object in"=w544, "error in (no error)"=w534) -> ("object out"=w541:refnum<class "Application.lvclass">, "CetoniPump"=w538:refnum<class "CetoniPump.lvclass">, "error out"=w540:errorcluster)  [unwired: 15 in]
        n214 = call-dynamic "SetFillLevel.vi"("object in"=w538, "GoToLevelSettings"=w531, "error in (no error)"=w540) -> ("object out"=w537:refnum<class "CetoniPump.lvclass">, "Coerced Level"=w536:dbl, "Coerced Flow"=w530:dbl, "error out"=w539:errorcluster)  [unwired: 12 in, 1 out]
        n215 = Bundle By Name(cluster=w531, "Level(ml)"=w536, "Flow"=w530) -> (w529:T4)
        n216 = call-dynamic "SetCetoniPump.vi"("object in"=w541, "CetoniPump"=w537, "error in (no error)"=w539) -> ("object out"=w543:refnum<class "Application.lvclass">, "error out"=w542:errorcluster)  [unwired: 15 in]
        n217 = local write "GoToLevelSettings"(w529) -> ()
      }
      frame "CetoniInit" {
        n218 = call-dynamic "GetCetoniPump.vi"("object in"=w556, "error in (no error)"=w555) -> ("object out"=w553:refnum<class "Application.lvclass">, "CetoniPump"=w552:refnum<class "CetoniPump.lvclass">, "error out"=w550:errorcluster)  [unwired: 15 in]
        n219 = call "CetoniPump_Init.vi"("object in"=w552, "Device Configuration Path"="Device Configuration Folder", "error in (no error)"=w550) -> ("object out"=w551:refnum<class "CetoniPump.lvclass">, "error out"=w549:errorcluster)  [unwired: 15 in]
        n220 = call-dynamic "SetCetoniPump.vi"("object in"=w553, "CetoniPump"=w551, "error in (no error)"=w549) -> ("object out"=w547:refnum<class "Application.lvclass">, "error out"=w554:errorcluster)  [unwired: 15 in]
        n221 = call-dynamic "FireUpdateStatus.vi"("object in"=w547, "Status"="Syringe Pump Initialized") -> ("object out"=w546:refnum<class "Application.lvclass">)  [unwired: 16 in, 1 out]
      }
      frame "CetoniReadStatus" {
        n222 = call-dynamic "GetCetoniPump.vi"("object in"=w569, "error in (no error)"=w566) -> ("object out"=w567:refnum<class "Application.lvclass">, "CetoniPump"=w565:refnum<class "CetoniPump.lvclass">, "error out"=w563:errorcluster)  [unwired: 15 in]
        n223 = call-dynamic "ReadStatusAllPumps.vi"("object in"=w565, "error in (no error)"=w563) -> ("object out"=w564:refnum<class "CetoniPump.lvclass">, "Array"=→"Pump Status":T1, "error out"=w562:errorcluster)  [unwired: 15 in]
        n224 = call-dynamic "SetCetoniPump.vi"("object in"=w567, "CetoniPump"=w564, "error in (no error)"=w562) -> ("object out"=w559:refnum<class "Application.lvclass">, "error out"=w568:errorcluster)  [unwired: 15 in]
        n225 = local read "Pump: Read Status"() -> (w557:bool)
        n226 = case shown="True" w557 {
          tunnel: "CetoniReadStatus" ("Message") -> [_ w573]
          tunnel: w559 -> [w570 w572]
          tunnel: [w570 w571] -> w558
          frame False {
          }
          frame True {
            n227 = call-dynamic "EnqueueMain.vi"("object in"=w572, "Message"=w573) -> ("object out"=w571:refnum<class "Application.lvclass">)  [unwired: 16 in, 1 out]
          }
        }
      }
      frame "CetoniReferenceMove" {
        n228 = call-dynamic "GetCetoniPump.vi"("object in"=w584, "error in (no error)"=w580) -> ("object out"=w581:refnum<class "Application.lvclass">, "CetoniPump"=w579:refnum<class "CetoniPump.lvclass">, "error out"=w576:errorcluster)  [unwired: 15 in]
        n229 = call-dynamic "GetConnectedPumps.vi"("object in"=w579) -> ("object out"=w578:refnum<class "CetoniPump.lvclass">, "ConnectedPumps"=w574:T16)  [unwired: 16 in, 1 out]
        n230 = for {
          shift-right: [w588] -> w577
          shift-left: w578 -> [w589]
          shift-right: [w586] -> w575
          shift-left: w576 -> [w587]
          tunnel: w574 -> [_] mode=indexing
          i -> [w585]
          n231 = call-dynamic "ReferenceMove.vi"("object in"=w589, "index"=w585, "error in (no error)"=w587) -> ("object out"=w588:refnum<class "CetoniPump.lvclass">, "error out"=w586:errorcluster)  [unwired: 15 in]
        }
        n232 = call-dynamic "SetCetoniPump.vi"("object in"=w581, "CetoniPump"=w577, "error in (no error)"=w575) -> ("object out"=w583:refnum<class "Application.lvclass">, "error out"=w582:errorcluster)  [unwired: 15 in]
      }
      frame "CetoniRefill" {
        n233 = Variant To Data(error in=w596, Variant=w598) -> (data=w591:i32, error out=w597:errorcluster)  [unwired: 1 in]
        n234 = call-dynamic "GetCetoniPump.vi"("object in"=w602, "error in (no error)"=w597) -> ("object out"=w599:refnum<class "Application.lvclass">, "CetoniPump"=w595:refnum<class "CetoniPump.lvclass">, "error out"=w593:errorcluster)  [unwired: 15 in]
        n235 = call-dynamic "Refill.vi"("object in"=w595, "Refill Rate"="Refill Rate(ul/min)", "index"=w591, "error in (no error)"=w593) -> ("object out"=w594:refnum<class "CetoniPump.lvclass">, "error out"=w592:errorcluster)  [unwired: 14 in]
        n236 = call-dynamic "SetCetoniPump.vi"("object in"=w599, "CetoniPump"=w594, "error in (no error)"=w592) -> ("object out"=w601:refnum<class "Application.lvclass">, "error out"=w600:errorcluster)  [unwired: 15 in]
      }
      frame "CetoniStopPumps" {
        n237 = call-dynamic "GetCetoniPump.vi"("object in"=w611, "error in (no error)"=w607) -> ("object out"=w608:refnum<class "Application.lvclass">, "CetoniPump"=w606:refnum<class "CetoniPump.lvclass">, "error out"=w604:errorcluster)  [unwired: 15 in]
        n238 = call-dynamic "StopAllPumps.vi"("object in"=w606, "error in (no error)"=w604) -> ("object out"=w605:refnum<class "CetoniPump.lvclass">, "error out"=w603:errorcluster)  [unwired: 16 in]
        n239 = call-dynamic "SetCetoniPump.vi"("object in"=w608, "CetoniPump"=w605, "error in (no error)"=w603) -> ("object out"=w610:refnum<class "Application.lvclass">, "error out"=w609:errorcluster)  [unwired: 15 in]
      }
      frame "Error" {
        # "#CodeRecommended - If you ever change the name of this \"Error\" message, you'll need to update the name in the Check Loop Error.vi as well."
        # "#CodeRecommended - Consider creating a system for logging errors in some way. These errors are for notification purposes only. Handling of specific errors should be performed in the message frames that generated the error."
        # "Error - Display an error dialog. This message is sent by the \"Error Handler\" VIs at the end of other loops in this application."
        n240 = Variant To Data(error in=w618, type=errorcluster {"status"=FALSE, "code"=0, "source"=""} ("error constant"), Variant=w617) -> (data=w615:errorcluster, error out=w614:errorcluster)
        n241 = call <vilib>:"Simple Error Handler.vi"("error in (no error)"=w615) -> ()  [unwired: 4 in, 5 out]
        n242 = Merge Errors(w614) -> (w613:errorcluster)
      }
      frame "Exit" {
        # "Stop the VI"
        # "Release the message queue reference"
        # "#CodeNeeded - Add any required cleanup code here. Note that if 'Exit' was called as a result of an error, an error dialog will be displayed. Add any custom error handling for an 'Exit' condition here as well."
        # "Exit - Exit the application."
        n243 = call <vilib>:"Simple Error Handler.vi"("error in (no error)"=w620) -> ("error out"=w619:errorcluster)  [unwired: 4 in, 4 out]
        n244 = call-dynamic "FireStopEvent.vi"("object in"=w622, "error in (no error)"=w619) -> ("object out"=w623:refnum<class "Application.lvclass">, "error out"=w621:errorcluster)  [unwired: 16 in]
      }
      frame "Initialize" {
        # "Initialize - All initialization work should take place in this message, since other loops can potentially enqueue messages that execute immediately after this one."
        n245 = Build Array("CoriolisInit", "CetoniInit", "HamamatsuInit", "AD2Init", "OscilloscopeInit" ("element"), "PeltierInit" ("element")) -> (w632:string[])
        n246 = for {
          shift-right: [w636] -> w630
          shift-left: w629 -> [w637]
          tunnel: w632 -> [w635] mode=indexing
          n247 = call-dynamic "EnqueueMain.vi"("object in"=w637, "Message"=w635) -> ("object out"=w636:refnum<class "Application.lvclass">)  [unwired: 16 in, 1 out]
        }
      }
      frame "MeasurePowerOsc" {
        n248 = call-dynamic "GetTBS2000.vi"("object in"=w647) -> ("object out"=w646:refnum<class "Application.lvclass">, "TBS2000Series"=w644:refnum<class "TBS2000Series.lvclass">)  [unwired: 16 in, 1 out]
        n249 = call-dynamic "Read Osc. Energy Density.vi"("object in"=w644, "Oscilloscope"="Oscilloscope Test", "milliseconds to wait"="milliseconds to wait 2", "error in (no error)"=w640) -> ("object out"=w643:refnum<class "TBS2000Series.lvclass">, "Oscilloscope Results"=→"Oscilloscope Results Test":T6, "error out"=w641:errorcluster)  [unwired: 9 in]
        n250 = call-dynamic "Set TBS2000.vi"("object in"=w646, "TBS2000Series"=w643) -> ("object out"=w645:refnum<class "Application.lvclass">)  [unwired: 16 in, 1 out]
      }
      frame "PeltierInit" {
        n251 = call-dynamic "GetTC0608.vi"("object in"=w653) -> ("object out"=w655:refnum<class "Application.lvclass">, "TC0608"=w657:refnum<class "TC0608.lvclass">)  [unwired: 16 in, 1 out]
        n252 = call "TC0608_Init.vi"("object in"=w657, "VISA resource name"="Peltier VISA resource name", "error in (no error)"=w650) -> ("object out"=w656:refnum<class "TC0608.lvclass">, "error out"=w651:errorcluster)  [unwired: 15 in]
        n253 = call-dynamic "SetTC0608.vi"("object in"=w655, "TC0608"=w656) -> ("object out"=w654:refnum<class "Application.lvclass">)  [unwired: 16 in, 1 out]
        n254 = call-dynamic "UpdateStatus.vi"("object in"=w654, "Status"="Peltier Initialized") -> ("object out"=w649:refnum<class "Application.lvclass">)  [unwired: 16 in, 1 out]
      }
      frame "PeltierRead" {
        n255 = call-dynamic "GetTC0608.vi"("object in"=w663) -> ("object out"=w665:refnum<class "Application.lvclass">, "TC0608"=w662:refnum<class "TC0608.lvclass">)  [unwired: 16 in, 1 out]
        n256 = call-dynamic "ReadTemperature.vi"("object in"=w662, "error in (no error)"=w660) -> ("object out"=w661:refnum<class "TC0608.lvclass">, "temperature (C)"=→"Temperature (C)":dbl, "error out"=w659:errorcluster)  [unwired: 15 in]
        n257 = call-dynamic "SetTC0608.vi"("object in"=w665, "TC0608"=w661) -> ("object out"=w664:refnum<class "Application.lvclass">)  [unwired: 16 in, 1 out]
      }
      frame "ReadOscilloscopeChannel" {
        n258 = call-dynamic "GetTBS2000.vi"("object in"=w671) -> ("object out"=w670:refnum<class "Application.lvclass">, "TBS2000Series"=w669:refnum<class "TBS2000Series.lvclass">)  [unwired: 16 in, 1 out]
        n259 = call-dynamic "Read Piezo Prefocus.vi"("object in"=w669, "Source (1: Channel 1)"="Source (1: Channel 1)") -> ("object out"=w668:refnum<class "TBS2000Series.lvclass">, "Frequency"=→"Frequency":dbl, "Peak-to-Peak"=→"Peak-to-Peak":dbl)  [unwired: 13 in, 2 out]
        n260 = call-dynamic "Set TBS2000.vi"("object in"=w670, "TBS2000Series"=w668) -> ("object out"=w672:refnum<class "Application.lvclass">)  [unwired: 16 in, 1 out]
      }
      frame "TakeNImages" {
        # "This Constants is set to give a 1ms pulse over 5ms span, pc triggered, and then wait for new trigger\nDo not Change unless you know how to set the DOs of the AD2"
        n261 = Variant To Data(error in=w678, type=T15 {"Minimum Time between frames"=10.0, "Number of Frames"=0} ("Image  Aquisition"), Variant=w681) -> (data=w677:T15, error out=w679:errorcluster)
        n262 = Unbundle By Name(w677) -> ("Minimum Time between frames"=w676:dbl, "Number of Frames"=w675:i32)
        n263 = call-dynamic "GetAD2_SDK.vi"("object in"=w685) -> ("object out"=w684:refnum<class "Application.lvclass">, "AD2_SDK"=w690:refnum<class "AD2_SDK.lvclass">, "error out"=w689:errorcluster)  [unwired: 16 in]
        n264 = call-dynamic "ConfigDO.vi"("object in"=w690, 2:T11 {"DO Trigger"={"secRun(0=Cont)"=0.005, "secWait"=0.0, "cRepeat(0=inf)"=0, "Repeat Trigger"=TRUE, "TrigrSrc"=enum."trigsrcPC"}, "CustomData"=[{"Data"=[FALSE, TRUE, FALSE, FALSE, FALSE, FALSE, FALSE, FALSE, FALSE, FALSE, FALSE, FALSE, FALSE, FALSE, FALSE, FALSE, FALSE, FALSE, FALSE, FALSE, FALSE, FALSE], "Freq"=1000.0, "#Bits"=100, "Enable"=TRUE, "IdleState"=0}, {"Data"=[], "Freq"=0.0, "#Bits"=0, "Enable"=FALSE, "IdleState"=0}, {"Data"=[], "Freq"=0.0, "#Bits"=0, "Enable"=FALSE, "IdleState"=0}, {"Data"=[], "Freq"=0.0, "#Bits"=0, "Enable"=FALSE, "IdleState"=0}, {"Data"=[], "Freq"=0.0, "#Bits"=0, "Enable"=FALSE, "IdleState"=0}, {"Data"=[], "Freq"=0.0, "#Bits"=0, "Enable"=FALSE, "IdleState"=0}, {"Data"=[], "Freq"=0.0, "#Bits"=0, "Enable"=FALSE, "IdleState"=0}, {"Data"=[], "Freq"=0.0, "#Bits"=0, "Enable"=FALSE, "IdleState"=0}, {"Data"=[], "Freq"=0.0, "#Bits"=0, "Enable"=FALSE, "IdleState"=0}, {"Data"=[], "Freq"=0.0, "#Bits"=0, "Enable"=FALSE, "IdleState"=0}, {"Data"=[], "Freq"=0.0, "#Bits"=0, "Enable"=FALSE, "IdleState"=0}, {"Data"=[], "Freq"=0.0, "#Bits"=0, "Enable"=FALSE, "IdleState"=0}, {"Data"=[], "Freq"=0.0, "#Bits"=0, "Enable"=FALSE, "IdleState"=0}]}, "error in (no error)"=w689) -> ("object out"=w687:refnum<class "AD2_SDK.lvclass">, "error out"=w688:errorcluster)  [unwired: 15 in]
        n265 = for {
          N: w675 -> [_]
          shift-right: [w695] -> w691
          shift-left: w688 -> [w700]
          shift-right: [w701] -> w692
          shift-left: w687 -> [w699]
          shift-right: [w697] -> w683
          shift-left: w684 -> [w698]
          tunnel: w676 -> [w693]
          stop <- w694 stop-if-true
          n266 = call-dynamic "PCTrig.vi"("object in"=w699, "error in (no error)"=w700) -> ("object out"=w701:refnum<class "AD2_SDK.lvclass">, "error out"=w696:errorcluster)  [unwired: 16 in]
          n267 = call-dynamic "Wait.vi"("object in"=w698, "Time to wait"=w693, "error in (no error)"=w696) -> ("object out"=w697:refnum<class "Application.lvclass">, "aborted"=w694:bool, "error out"=w695:errorcluster)  [unwired: 14 in]
        }
        n268 = call-dynamic "SetAD2_SDK.vi"("object in"=w683, "AD2_SDK"=w692, "error in (no error)"=w691) -> ("object out"=w686:refnum<class "Application.lvclass">)  [unwired: 15 in, 1 out]
      }
      frame "Wait" {
        n269 = Variant To Data(error in=w710, Variant=w712) -> (data=w711:dbl, error out=w707:errorcluster)  [unwired: 1 in]
        n270 = call-dynamic "FireUpdateStatus.vi"("object in"=w708, "Status"="waiting.....") -> ("object out"=w705:refnum<class "Application.lvclass">)  [unwired: 16 in, 1 out]
        n271 = call-dynamic "Wait.vi"("object in"=w705, "Time to wait"=w711, "error in (no error)"=w707) -> ("object out"=w709:refnum<class "Application.lvclass">, "error out"=w706:errorcluster)  [unwired: 14 in, 1 out]
        n272 = call-dynamic "FireUpdateStatus.vi"("object in"=w709, "Status"="wait complete") -> ("object out"=w703:refnum<class "Application.lvclass">)  [unwired: 16 in, 1 out]
      }
      frame Default {
        # "'Default' case only runs if there is a message that isn't defined in any of the other cases.  Output a programming error."
        n273 = xnode "Error Ring"("parameter 0"=w714) -> ("error out"=w715:errorcluster)
      }
    }
    n274 = call-dynamic "ErrorHandlerMainLoop.vi"("object in"=w192, "error in (no error)"=w195) -> ("object out"=w193:refnum<class "Application.lvclass">, "error out"=w194:errorcluster)  [unwired: 16 in]
  }
  n275 = Merge Errors(w5, w6) -> (w4:errorcluster)
  n276 = call-dynamic "CleanUp.vi"("object in"=w7, "error in (no error)"=w4) -> ("error out"=→"error out":errorcluster)  [unwired: 16 in, 1 out]
